vi "App - temperature sweep P1.vi"() -> ()   [LabVIEW 2014]
uses:
  C:/Users/riggslab/Desktop/Paula/maglab ultrasound -- arkady_by20151113_modified/state.ctl
  C:/Users/riggslab/Desktop/Paula/maglab ultrasound -- arkady_by20151113_modified/Sample_Temperature_Source_Control.ctl
  save log.ctl
  RUS/Controls/Sweep settings.ctl
  RUS/Controls/Lock-in DAQ settings.ctl
  File/Controls/Save data settings.ctl
  File/Controls/File formats.ctl
  C:/Users/riggslab/Desktop/Paula/maglab ultrasound -- arkady_by20151113_modified/ITC Panel.ctl
  gas flow controller control.ctl
  gas flow control - progress.ctl
  alarm clock control.ctl
  temperature indicator.ctl
  adaptive sweep UI controls.ctl
  next chunk -- algorithm.ctl
  time in gamma mode control.ctl
  Set Temperature PID - Control.ctl
  Scott -- strain -- strain sweep control.ctl
  FSU/ScottRiggs/Piezo2/voltage-wave-generator-parameters.ctl
  pair.ctl
  ctl -- name dispatcher -- action.ctl
  p9action control.ctl
  countdown control.ctl
  gas flow controller action.ctl
  C:/Users/riggslab/Desktop/Paula/maglab ultrasound -- arkady_by20151113_modified/itc 503 box - control.ctl
  Instruments/Neocera/Neocera Set Point Aproach.ctl
  file -- 9w path.vi
  Q - not nan -- real.vi
  Q - not nan and gtr than zero.vi
  switch - C.vi
  aggregator - ii - real.vi
  linear interpolation.vi
  <vilib>/Utility/libraryn.llb/Check if File or Folder Exists.vi
  file -- scan filename logic -- V1.vi
  <vilib>/Utility/file.llb/Write To Spreadsheet File.vi
  <vilib>/Utility/file.llb/Write To Spreadsheet File (string).vi
  <vilib>/regexp/Match Regular Expression.xnode
  Scott -- strain -- sweep parameter action.ctl
panel:
  in  "sweep folder path":path=path "D:/Technique/RUS/URuSi/DU45-325/2_cooling"
  in  "Tab: everything":T1(tab)=enum."temperature" caption="Tab Control"
  in  "Tab: RUS controls":T2(tab)
  in  "RUS settings":enum32{"main", "save and staff"}(tab)
  in  "adaptive sweep settings":T3={"time gap (min) "=0.0, "Bypass error dialog"=TRUE, "range factor"=1.35, "min gamma(kHz)"=0.005, "max step(Hz)"=1500.0, "min step(Hz)"=0.001, "save freq units"=enum."kHz", "Zero signal?"=FALSE, "time in Gamma --OK"=TRUE, "scan mode"=enum."peak position is known", "power control mode "=enum."none", "time-in-gamma mode"=enum."same for all"}
  in  "Lock-in DAQ settings":T6={"Lockin mode"=enum."NI-DAQ", "DAQmx Device"="Dev2", "SR Lockin"="GPIB0::10::INSTR", "Clock Multiplier"=64, "Low-pass filter"=enum."No filtering", "Ranges and couplings "=[{"Range"=2.5, "Coupling"=10106}], "Samples per read"=20, "Record IF"=FALSE, "Auto-phase"=FALSE} {"Ranges and couplings"."Coupling" items=["default"=-1, "RSE"=10083, "NRSE"=10078, "Differential"=10106, "Pseudodifferential"=12529]}
  in  "Fast sweep settings":T7={"Update rate (Hz)"=200.0, "Start F, Hz"=100000.0, "Stop F"=3500000.0, "Number of points"=7290, "Amplitude"=0.7, "Init&amplitude"=TRUE, "IF"=1000.0, "Time constant"=0.001} {"IF" format="%#_6p"; "Amplitude" min=0.0 max=2.5; "Number of points" format="%.0p"; "Stop F" format="%#_6p"; "Start F, Hz" format="%#_6p"; "Update rate (Hz)" format="%0.2f"}
  in  "Save data settings":T8={"Save data"=TRUE, "Data Root Path"=path "D:/Technique/RUS/URuSi/DU45-325/2_cooling", "File Prefix"="298.56700K_100_3500_0.70000V_0.00000T_Jul13-2015__11-06-01_", "File Format"=enum."BINARY", "Save column names"=FALSE, "File Comments"="\r\nColumns:Frequency\\tX\\tY\r\n    ITC Temp= 299.200000\r\n    LTC Temp= 0.000000\r\n          ITC_set=295.00000\r\n", "User/Prj"="<User Name/Project Description>"}
  out "sweep time  (min)":dbl=3.3333333333333335
  out "sweep time (sec)":i32=200
  out "kHz/second":dbl=17.0
  in  "RUS loop":bool=TRUE
  in  "RUS zeroed":bool
  in  "read AH every # sec":dbl=1.7
  in  "plot":T10(ring)=enum."Capac vs Temp"
  out "temperature":dbl=198.969
  out "time(min)":dbl
  out "Capacitance":dbl=0.600435
  out "Loss":dbl=0.00206
  in  "save every # (min)":dbl=7.12
  in  "history length (min)":dbl=60.0
  in  "Sweep folder path":path=path "C:/data/RUS/Experiment/ProbeTest/cantilever/Hg1201-2-2/sweep1"
  in  "VISA - AH2500":refnum<visa-resource-name>="GPIB0::28::INSTR"
  in  "take cantilever reading":bool=TRUE
  out "Plot: capacitance":cluster{dbl[], dbl[]}[](graph)
  in  "plot lever  ?":bool
  in  "Strain Inner Tabs":enum32{"Other", "Main"}(tab)=enum."Main"
  in  "time gap (min)":dbl
  in  "strain sweep control":T11={"just in case"=TRUE, "Piezo Amplifier settings"={"Gain "=69.44, "offset (V)"=-50.0}, "voltage-parameters-IN"={"phase "=0.7853981633974483, "amplitude (V)"=2.8801843317972353, "offset (V)"=0.0, "time delay (sec)"=0.5, "period (sec)"=50.0, "shape"=enum."triangle"}, "Lockin Settings"=[{"Offset"=FALSE, "GPIB Address"=6}, {"Offset"=TRUE, "GPIB Address"=7}], "VISA address Agilent  IN"="GPIB0::22::INSTR", "number of iterations"=1.0, "Piezo sweep settings"={"max Piezo voltage (V) "=150.0, "min Piezo voltage (V)"=-50.0, "delay (sec)"=0.5, "period (sec)"=50.0, "shape"=enum."triangle"}}
  in  "Strain loop":bool
  in  "show plot pallets":bool
  in  "Tab: ITC controls":enum32{"display", "gas ", "progress"}(tab)
  in  "set  T target":T13(ring)=enum."set T -> ITC (oxford)"
  in  "Set Temperature PID":T14={"mode "=enum."bezier", "set temperature?"=FALSE, "Time(min)"=646.03001, "Temperature(K)"=251.5695804259867, "OK?"=TRUE, "interval(sec)"=3.1}
  in  "ITC panel":T15={"Locked"=TRUE, "Unlocked"=FALSE, "Remote"=FALSE, "Local"=TRUE, "in sweep"=FALSE, "start/stop sweep"=FALSE, "Sweep indicator"="NOT in sweep", "heater MANUAL"=TRUE, "heater AUTO"=FALSE, "ITC state"="X0A1C2S01H1L0\r", "gas MANUAL"=TRUE, "gas AUTO"=FALSE, "heater"=5.999, "gas flow %"=20.587} {"gas flow %" format="%.3g"; "heater" format="%.3g"}
  in  "itc box: set temperature to: value":dbl=295.0
  in  "set temperature to":bool
  in  "disable interaction with itc":T16(ring)
  in  "plot?":bool=TRUE
  in  "set heater to":bool
  in  "itc box: set heater to: value":dbl=7.0
  in  "gas flow controller":T17={"DOWN step (%)"=0.5, "below"=FALSE, "above"=FALSE, "check (min)"=3.0, "upper"=12.0, "lower"=5.0, "in range"=TRUE, "ramp step (%)"=0.1, "DOWN time (min)"=20.0, "UP time (min)"=20.0, "UP step (%)"=0.5, "set gas"=FALSE, "to"=20.0, "ramp UP"=FALSE, "ramp DOWN"=FALSE, "idle"=TRUE, "Control Gas"=TRUE, "state"=enum."normal", "ramp Up progress"={"(total # of ramp steps)"=5, "ramp time step (sec)"=240, "steps so far"=0, "state"=enum."normal"}, "ramp Down progress"={"(total # of ramp steps)"=5, "ramp time step (sec)"=240, "steps so far"=0, "state"=enum."normal"}, "last (min)"=1.4983333333333335, "heater"=5.9990000000000085, "gas, %"=20.587} {"last (min)" format="%3.3f"}
  out "ramp Down progress":T18={"(total # of ramp steps)"=5, "ramp time step (sec)"=240, "steps so far"=0, "state"=enum."normal"}
  out "ramp Up progress":T18={"(total # of ramp steps)"=5, "ramp time step (sec)"=240, "steps so far"=0, "state"=enum."normal"}
  in  "Tab: plots":enum32{"Plot:  gas/heater", "Plot: temperayre"}(tab)=enum."Plot: temperayre"
  out "Plot: heater/gas":cluster{dbl[], dbl[]}[](graph)
  out "Plot: temperature":cluster{dbl[], dbl[]}[](graph)
  in  "Tab: controls":enum32{"indicators", "counter", "boxes"}(tab)
  in  "temperature indicator panel":T19={"LTC T"=298.568, "ITC T"=296.823, "ITC Set T"=296.82, "LTC T slope, K/min"=-0.0031198686372143165, "heater i-average, V"=5.999000000000011, "heater slope, V/min"=1.6517122458476368e-14, "LTC T i-average, K"=298.56648412698405, "ITC T i-average, K"=-2.7308309131347598e-14, "gas"=0.0} {"ITC Set T" format="%.3g"; "ITC T" format="%.3g"; "LTC T" format="%.3g"; "gas" format="%.3g"; "ITC T i-average, K" format="%#.5f"; "LTC T i-average, K" format="%#.5f"; "heater i-average, V" format="%.3g"; "heater slope, V/min" format="%#.5f"; "LTC T slope, K/min" format="%#.5f"}
  in  "Tab : everything to zero":enum32{"Page 1", "Page 2"}(tab)
  in  "alarm":T20={"counter (min)"=0.0, "alarm"=FALSE, "start"=FALSE, "set (min)"=1600.0, "stop"=FALSE} {"set (min)" format="%_4f"; "counter (min)" format="%_4f"}
  in  "Tab : Overheat":enum32{"Page 1"}(tab)
  in  "Over heat Temperature":dbl=315.0
  in  "Overheat protection":bool
  in  "Overheat !!":bool
  in  "temperature boxes":T21={"LTC21 Address"="GPIB0::15::INSTR", "ITC503 Address"="GPIB0::1::1::INSTR", "ITC temperature"=296.823, "ITC set temperature"=296.82, "LTC temperature"=298.568, "heater"=5.999, "gas flow"=20.587, "P"=6.5, "D"=0.0, "I"=0.9, "ITC state"="", "nonzero temperature"=298.568, "Magn Field (T)"=0.0, "LakeShore340"="GPIB0::11::INSTR", "LS340 Adress"=11, "Sample Temperature Source"=enum."read T <- LakeShore 340", "Neocera sensor"=1}
  in  "PID timer":dbl(slide)=86.6820000000298 min=-85661543.0 max=2135380277.0 step=0.010000000000000002 scale=0.0..100.0 scale format="%#3_3f"
  out "PID OK":bool=TRUE
  out "PID":dbl[](array[numeric])=[9.448275387987417, 0.584305003790149, 0.1]
  out "PID temperature":dbl=296.823
  out "Uploading ...":bool
  in  "Tab : Upload Sweep table":enum32{"Page 1"}(tab)
  out "Sweep Rates , min/K":dbl[](array[numeric])=[12.0, -0.0, 0.0, 0.0, 0.0, 0.0, 0.0, 0.0, 0.0, 0.0, 0.0, 0.0, 0.0, 0.0, 0.0, 0.0]
  out "current set temperature":dbl=50.0
  in  "set temperature":dbl=295.0
  in  "new sweep table":dbl[][](array[numeric])=[[200.0, 1000.0, 0.0], [100.0, 500.0, 0.0], [0.0, 0.0, 0.0], [0.0, 0.0, 0.0], [0.0, 0.0, 0.0], [0.0, 0.0, 0.0], [0.0, 0.0, 0.0], [0.0, 0.0, 0.0], [0.0, 0.0, 0.0], [0.0, 0.0, 0.0], [0.0, 0.0, 0.0], [0.0, 0.0, 0.0], [0.0, 0.0, 0.0], [0.0, 0.0, 0.0], [0.0, 0.0, 0.0], [70.0, 0.0, 0.0]]
  in  "Read Sweep Table in the box":bool
  out "Sweep Table":dbl[][](array[numeric])=[[70.0, 240.0, 1000.0], [0.0, 0.0, 0.0], [0.0, 0.0, 0.0], [0.0, 0.0, 0.0], [0.0, 0.0, 0.0], [0.0, 0.0, 0.0], [0.0, 0.0, 0.0], [0.0, 0.0, 0.0], [0.0, 0.0, 0.0], [0.0, 0.0, 0.0], [0.0, 0.0, 0.0], [0.0, 0.0, 0.0], [0.0, 0.0, 0.0], [0.0, 0.0, 0.0], [0.0, 0.0, 0.0], [70.0, 0.0, 0.0]]
  in  "upload new sweep table":bool
  out "index":dbl[][](array[numeric])=[[0.0, 1200.0, 0.0], [1.0, 1200.0, 0.0], [2.0, 500.0, 0.0], [3.0, 1399.0, 0.0], [4.0, 10.0, 1399.0], [5.0, 10.0, 1399.0], [6.0, 0.0, 0.0], [7.0, 0.0, 0.0], [8.0, 0.0, 0.0], [9.0, 0.0, 0.0], [10.0, 0.0, 0.0], [11.0, 0.0, 0.0], [12.0, 0.0, 0.0], [13.0, 0.0, 0.0], [14.0, 0.0, 0.0], [15.0, 0.0, 0.0]]
  out "date string Array":string[](array[string])=["Fri, Mar 07, 2014   :   11:06 AM", "Fri, Mar 07, 2014   :   3:06 PM"]
  in  "Rates , min/K":dbl[](array[numeric])=[12.0, -0.0, 0.0, 0.0, 0.0, 0.0, 0.0, 0.0, 0.0, 0.0, 0.0, 0.0, 0.0, 0.0, 0.0, 0.0]
  in  "use":bool
  out "writing log to":string="E:\\data\\Ultrasound\\Experiment\\ProbeTest\\Birdcage\\saphire-test\\1_test\\itc_log\\Stability_101113.dat"
  out "log line":string="time=Oct11,2013__13:45:08\tLTC=0.00000\tITC=0.00000\t ITC_set=0.00000\t\t filename=300.00000K_200_1000_2.10000V_0.00000T_Oct11-2013__13-45-08_101113.dat\t"
  out "saving log to":string
  out "saving sweep table to":string
  in  "save log":T23={"file path"=path "E:/data/Ultrasound/Experiment/ProbeTest/Birdcage/saphire-test/1_test", "Save log?"=TRUE, "every # of sec"=64}
  in  "set gas % to":dbl=10.0
  out "9ctl OK":bool
  out "minutes":dbl=1.4983333333333335
  out "milliseconds per cycle":u32=3100
  out "seconds per cycle":dbl=3.1
  out "file name prefix":string="298.56700K_100_3500_0.70000V_0.00000T_Jul13-2015__11-06-01_"
  out "x-y":dbl=37.2
  out "seconds":dbl=89.9
  in  "error in":errorcluster
  # "1. Make sure the correct experiment is hard-wired in the block diagram.\n2. Folder with 9w sub-folder. \n3. Reset ctl_set_temperature_TIMER file to 0.\n4. Set-up the ctl_set_temperature file."
  # "69.44"
  # "the paths are copied from \"data root path\" in the first page"
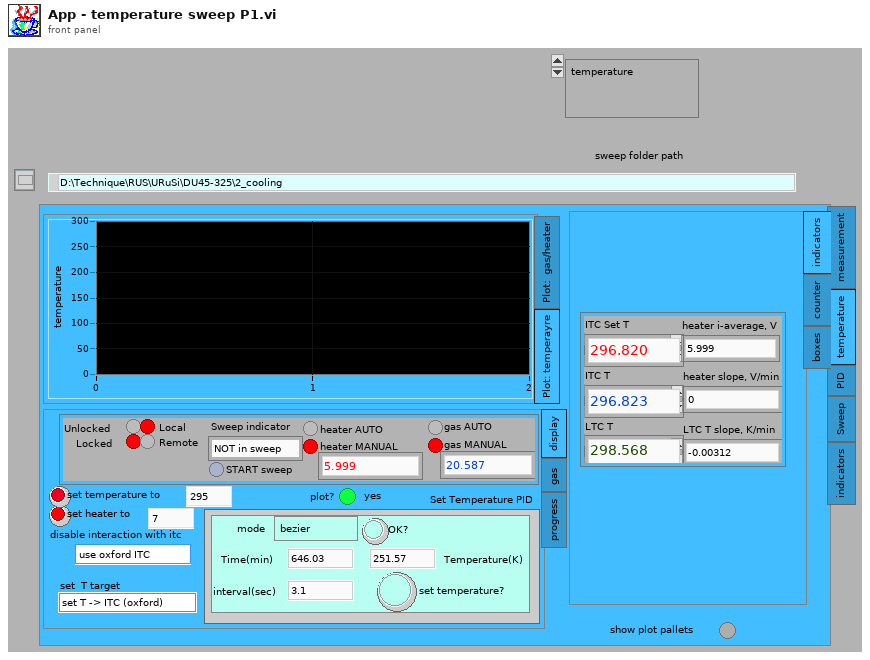
[diagram p1: front panel]
types:
  T1 = enum32{"measurement", "temperature", "PID", "Sweep", "indicators"}
  T2 = enum32{"Resonant Ultrasound", "Cantilever", "Strain"}
  T3 = typedef "adaptive sweep UI controls.ctl" = cluster{"time gap (min) ":dbl, "Bypass error dialog":bool, "range factor":dbl, "min gamma(kHz)":dbl, "max step(Hz)":dbl, "min step(Hz)":dbl, "save freq units":enum16{"kHz", "Hz"}, "Zero signal?":bool, "time in Gamma --OK":bool, "scan mode":T4, "power control mode ":enum16{"power vs Temp", "power vs Time", "none"}, "time-in-gamma mode":T5}
  T4 = typedef "next chunk -- algorithm.ctl" = enum16{"peak position is known", "uniform", "predictive"}
  T5 = typedef "time in gamma mode control.ctl" = enum16{"same for all", "each one different", "uniform scan"}
  T6 = typedef "Lock-in DAQ settings.ctl" = cluster{"Lockin mode":enum16{"SRS", "NI-DAQ"}, "DAQmx Device":tag, "SR Lockin":refnum<visa-resource-name>, "Clock Multiplier":i32, "Low-pass filter":enum16{"No filtering", "Butterworth", "Bessel"}, "Ranges and couplings ":cluster{"Range":dbl, "Coupling":i32}[], "Samples per read":i32, "Record IF":bool, "Auto-phase":bool}
  T7 = typedef "Sweep settings.ctl" = cluster{"Update rate (Hz)":dbl, "Start F, Hz":dbl, "Stop F":dbl, "Number of points":i32, "Amplitude":dbl, "Init&amplitude":bool, "IF":dbl, "Time constant":dbl}
  T8 = typedef "Save data settings.ctl" = cluster{"Save data":bool, "Data Root Path":path, "File Prefix":string, "File Format":T9, "Save column names":bool, "File Comments":string, "User/Prj":string}
  T9 = typedef "File formats.ctl" = enum16{"TDMS", "ASCII", "BINARY"}
  T10 = enum16{"Capac vs Time", "Capac vs Temp", "Loss  vs Time", "Loss vs Temp", "Delta Cap vs Temp"}
  T11 = typedef "Scott -- strain -- strain sweep control.ctl" = cluster{"just in case":bool, "Piezo Amplifier settings":cluster{"Gain ":dbl, "offset (V)":dbl}, "voltage-parameters-IN":T12, "Lockin Settings":cluster{"Offset":bool, "GPIB Address":i16}[], "VISA address Agilent  IN":refnum<visa-resource-name>, "number of iterations":dbl, "Piezo sweep settings":cluster{"max Piezo voltage (V) ":dbl, "min Piezo voltage (V)":dbl, "delay (sec)":dbl, "period (sec)":dbl, "shape":enum16{"triangle", "sine", "none"}}}
  T12 = typedef "voltage-wave-generator-parameters.ctl" = cluster{"phase ":dbl, "amplitude (V)":dbl, "offset (V)":dbl, "time delay (sec)":dbl, "period (sec)":dbl, "shape":enum16{"triangle", "sine", "none"}}
  T13 = enum16{"set T -> LTC (neocera)", "set T -> ITC (oxford)"}
  T14 = typedef "Set Temperature PID - Control.ctl" = cluster{"mode ":enum16{"bezier", "sine wave"}, "set temperature?":bool, "Time(min)":dbl, "Temperature(K)":dbl, "OK?":bool, "interval(sec)":dbl}
  T15 = typedef "ITC Panel.ctl" = cluster{"Locked":bool, "Unlocked":bool, "Remote":bool, "Local":bool, "in sweep":bool, "start/stop sweep":bool, "Sweep indicator":string, "heater MANUAL":bool, "heater AUTO":bool, "ITC state":string, "gas MANUAL":bool, "gas AUTO":bool, "heater":dbl, "gas flow %":dbl}
  T16 = enum16{"use oxford ITC", "do not use oxford ITC"}
  T17 = typedef "gas flow controller control.ctl" = cluster{"DOWN step (%)":dbl, "below":bool, "above":bool, "check (min)":dbl, "upper":dbl, "lower":dbl, "in range":bool, "ramp step (%)":dbl, "DOWN time (min)":dbl, "UP time (min)":dbl, "UP step (%)":dbl, "set gas":bool, "to":dbl, "ramp UP":bool, "ramp DOWN":bool, "idle":bool, "Control Gas":bool, "state":enum16{"normal", "ramp up", "ramp down"}, "ramp Up progress":T18, "ramp Down progress":T18, "last (min)":dbl, "heater":dbl, "gas, %":dbl}
  T18 = typedef "gas flow control - progress.ctl" = cluster{"(total # of ramp steps)":i32, "ramp time step (sec)":i32, "steps so far":i32, "state":enum16{"normal", "ramp up", "ramp down"}}
  T19 = typedef "temperature indicator.ctl" = cluster{"LTC T":dbl, "ITC T":dbl, "ITC Set T":dbl, "LTC T slope, K/min":dbl, "heater i-average, V":dbl, "heater slope, V/min":dbl, "LTC T i-average, K":dbl, "ITC T i-average, K":dbl, "gas":dbl}
  T20 = typedef "alarm clock control.ctl" = cluster{"counter (min)":dbl, "alarm":bool, "start":bool, "set (min)":dbl, "stop":bool}
  T21 = typedef "state.ctl" = cluster{"LTC21 Address":refnum<visa-resource-name>, "ITC503 Address":refnum<visa-resource-name>, "ITC temperature":dbl, "ITC set temperature":dbl, "LTC temperature":dbl, "heater":dbl, "gas flow":dbl, "P":dbl, "D":dbl, "I":dbl, "ITC state":string, "nonzero temperature":dbl, "Magn Field (T)":dbl, "LakeShore340":refnum<visa-resource-name>, "LS340 Adress":i16, "Sample Temperature Source":T22, "Neocera sensor":i32}
  T22 = typedef "Sample_Temperature_Source_Control.ctl" = enum16{"read T <- LakeShore 340", "read T <- Neocera"}
  T23 = typedef "save log.ctl" = cluster{"file path":path, "Save log?":bool, "every # of sec":i32}
  T24 = typedef "pair.ctl" = cluster{"num":i32, "bool":bool, "string":string}
  T25 = typedef "ctl -- name dispatcher -- action.ctl" = enum16{"peak frequency", "peak frequency DUMP", "peak gamma DUMP", "peak gamma", "peak frequency TEST", "peak gamma TEST", "ultrasonic power", "time in gamma", "set temperature ", "set temperature timer", "peak default gamma", "last scan file", "peak freq gamma TEST", "peak NAMES", "errors", "P_I_D", "P", "I", "D", "power vs time", "power vs time TIMER", "void", "power log", "set temperature - SINE", "itc ltc log", "peak - time in gamma"}
  T26 = typedef "Scott -- strain -- sweep parameter action.ctl" = enum16{"calculate gain and stuff", "none"}
  T27 = typedef "file -- scan filename.ctl" = cluster{"mmddyy (str)":string, "counter (str)":string, "to F (kHz)":dbl, "from F (kHz)":dbl, "temperature (K)":dbl, "date/time string":string, "time stamp":timestamp, "base name":string, "temperature (str)":string, "from F (str)":string, "to F (str)":string, "format":enum16{"no date string", "with date string"}, "power (V)":dbl, "power (str) ":string, "Magn Field (T)":dbl, "Magn Field (str)":string}
  T28 = cluster{"temperature array":dbl[], "delta capacitance array":dbl[]}
  T29 = cluster{"temperature array":dbl[], "delta capacitance array":dbl[]}[]
  T30 = typedef "p9action control.ctl" = enum16{"init", "check", "reset", "log", "message", "change path"}
  T31 = typedef "countdown control.ctl" = enum16{"check", "start", "reset cont", "stop", "reset once"}
  T32 = typedef "gas flow controller action.ctl" = enum16{"check", "force UP", "stop UP/DOWN", "force DOWN", "init", "set gas to", "turn off", "turn on", "idle", "update parameters", "parse", "set gas"}
  T33 = typedef "itc 503 box - control.ctl" = enum16{"heater manual and zero", "heater auto", "upload D", "upload I", "upload P", "shut off", "init", "read sweep table", "disable", "enable", "read state", "set gas to", "stop sweep", "start sweep", "test", "set temperature to", "write sweep table", "-void", "set heater to"}
  T34 = enum16{"table to rates", "rates to table", "other"}
  T35 = enum16{"parse", "start sweep", "stop sweep", "heater auto", "heater manual", "set heater"}
  T36 = enum8{"Enabled", "Disabled", "Disabled and Grayed Out"}
  T37 = typedef "Neocera Set Point Aproach.ctl" = enum16{"Instant", "Ramp"}
  T38 = typedef "itc 503 box state.ctl" = cluster{"ITC503 Address":refnum<visa-resource-name>, "ITC temperature":dbl, "ITC set temperature":dbl, "heater":dbl, "gas flow":dbl, "P":dbl, "D":dbl, "I":dbl, "ITC state":string, "nonzero temperature":dbl, "Magn Field (T)":dbl}
  T39 = enum16{"check", "force UP", "stop UP/DOWN", "force DOWN", "init", "set gas to", "turn off", "turn on", "update parameters"}
  T40 = enum32{"Page Enabled", "Page Disabled", "Page Disabled & Grayed"}
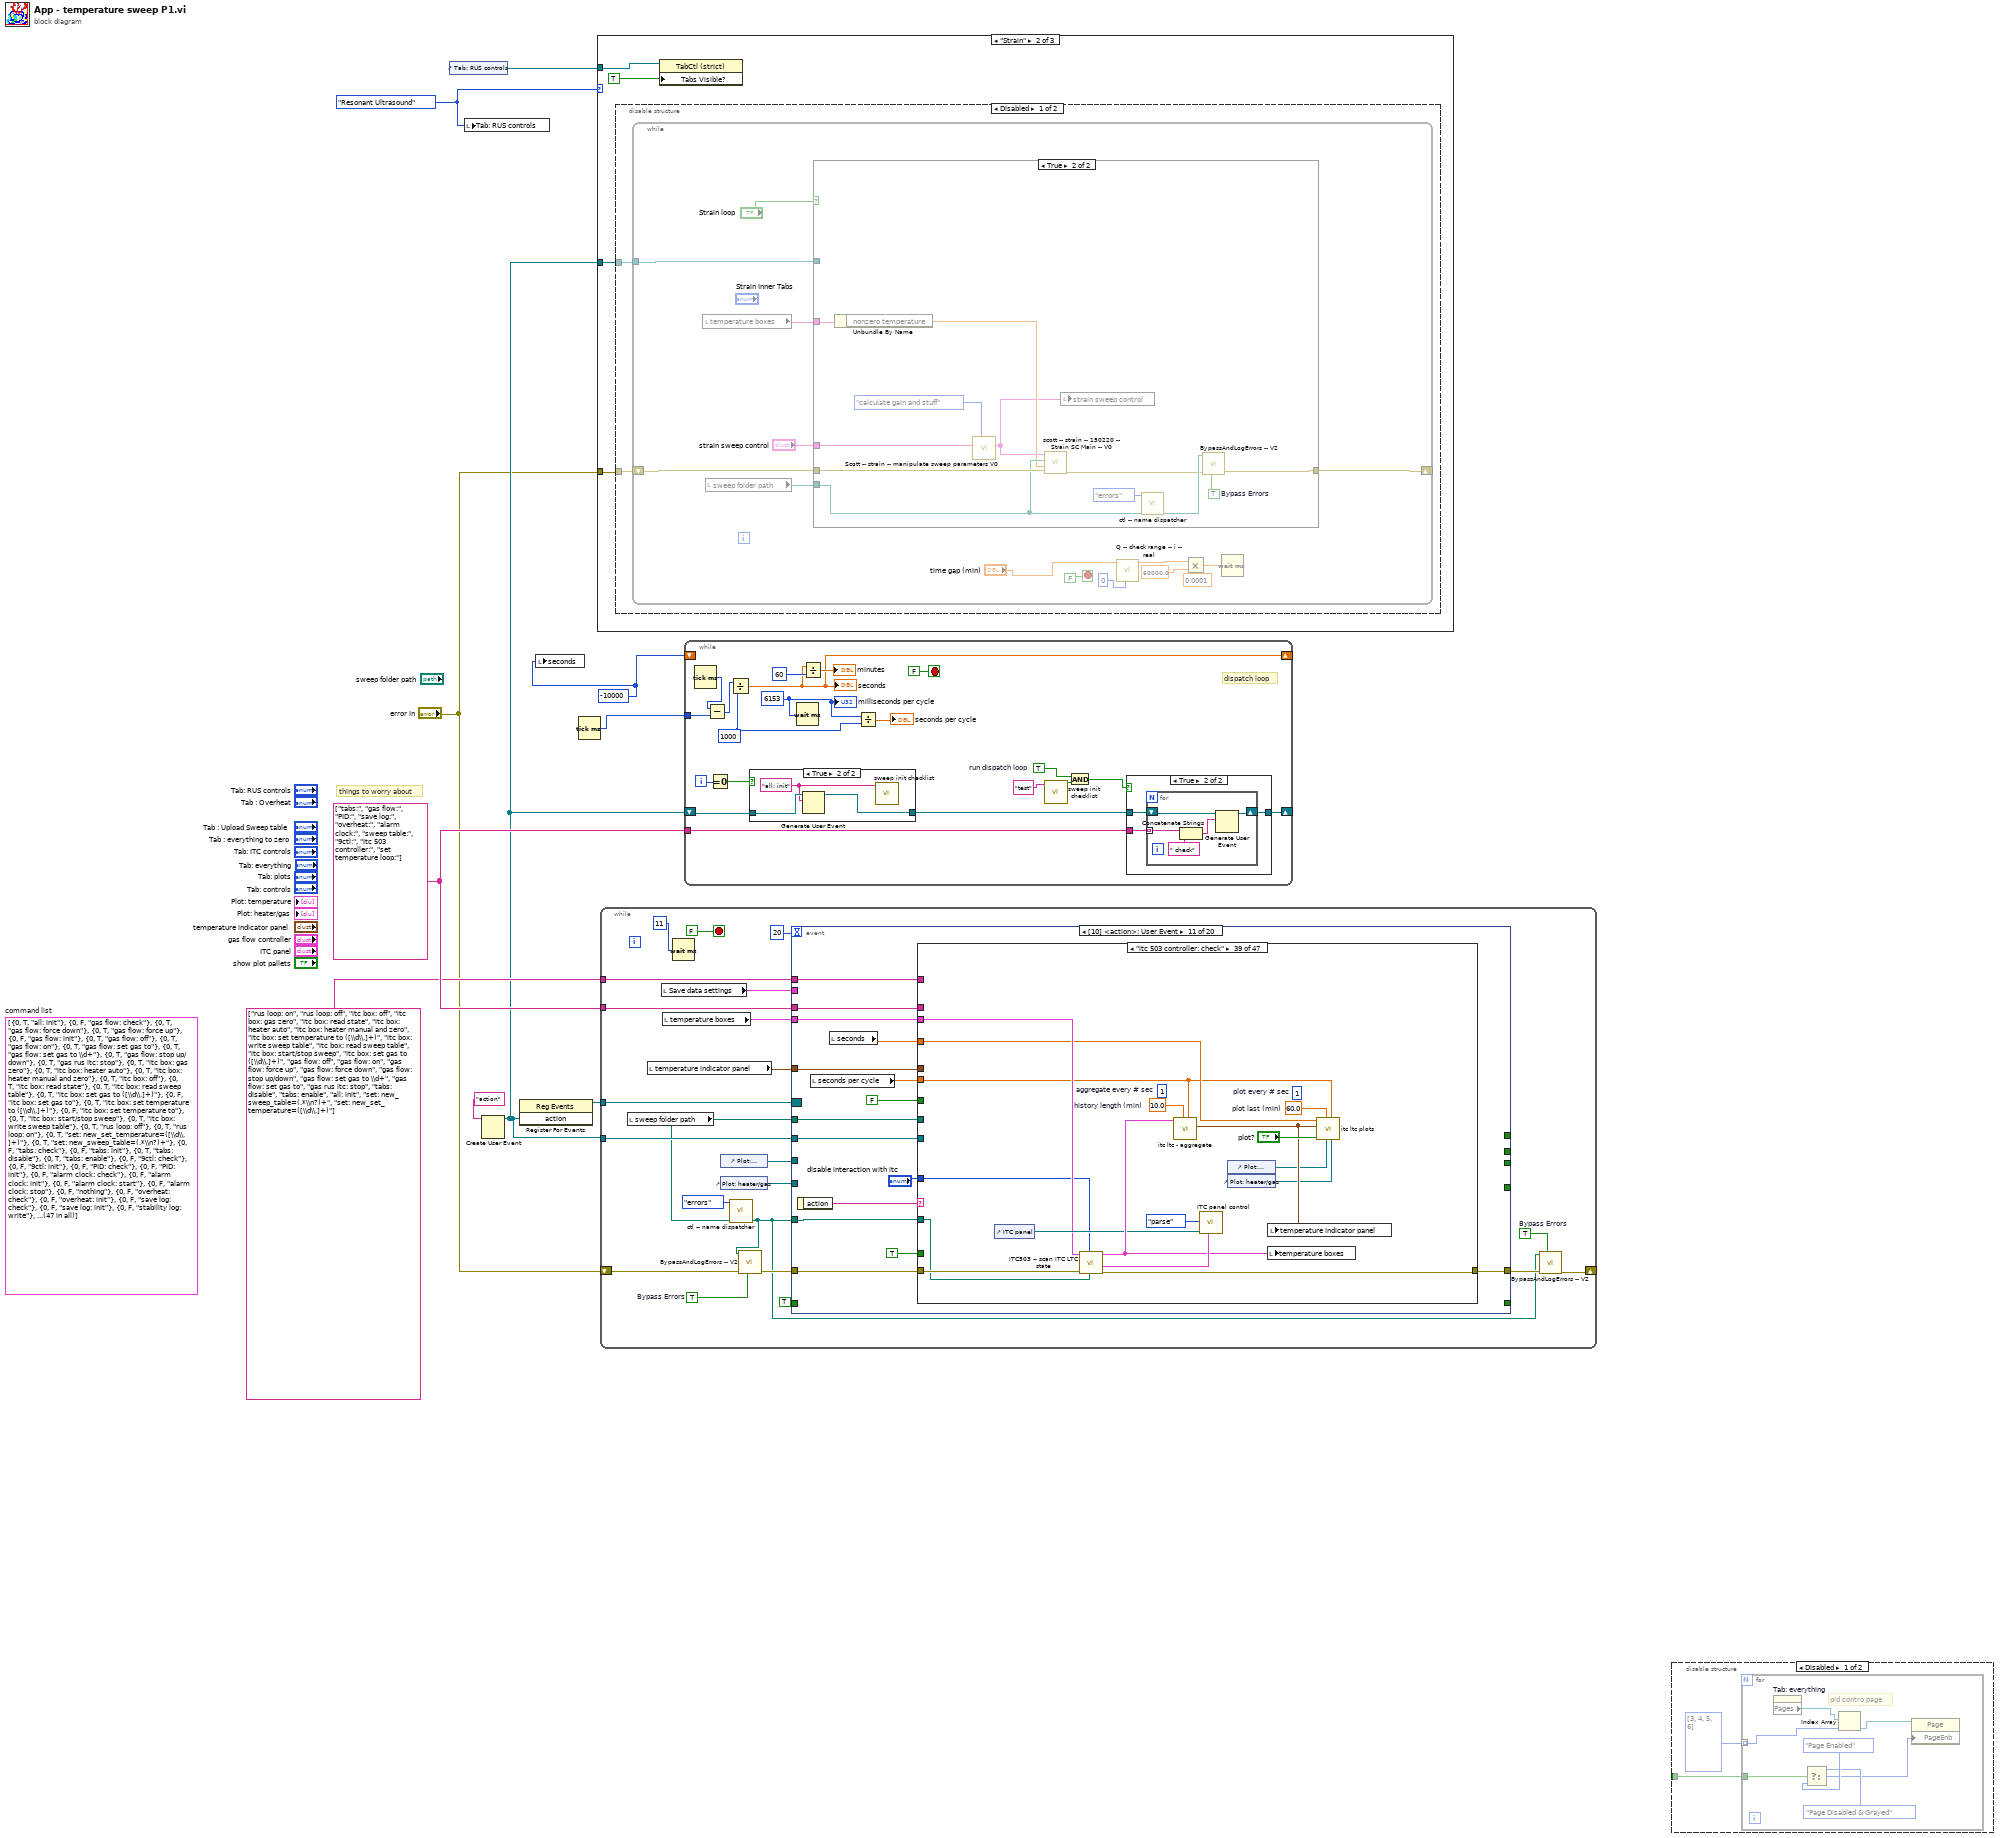
[diagram p0: block diagram]
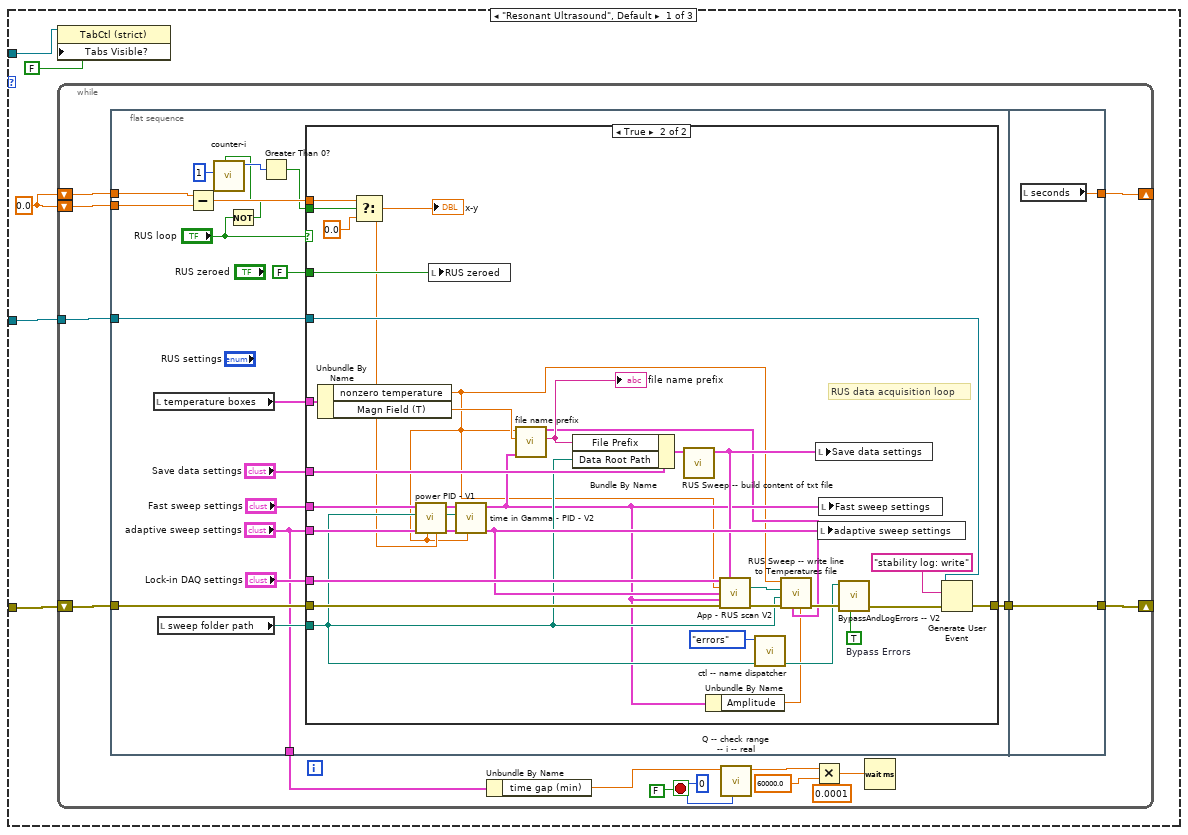
[diagram p2: hidden frame]
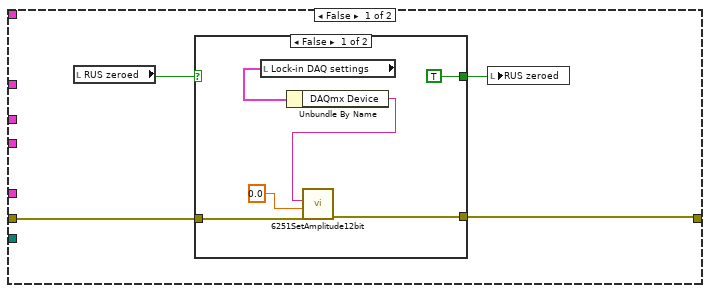
[diagram p3: hidden frame]
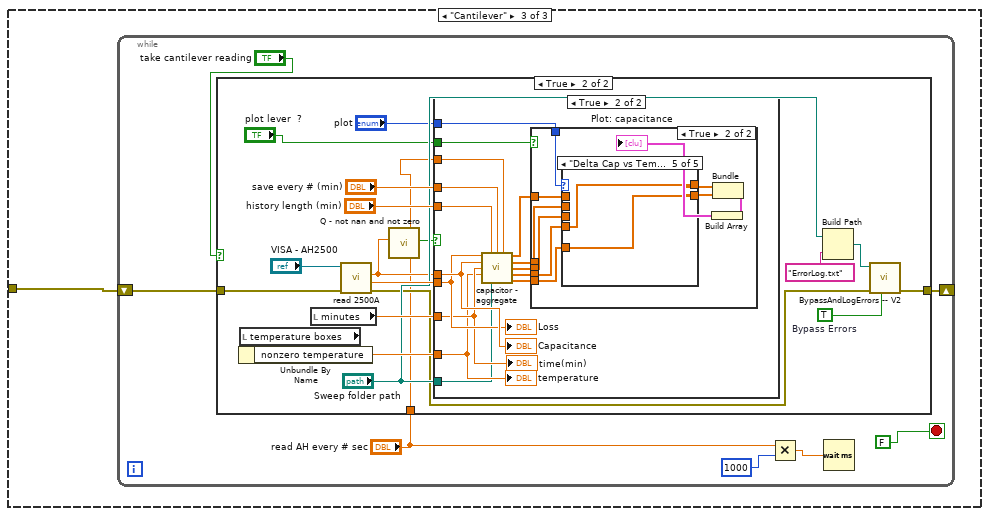
[diagram p7: hidden frame]
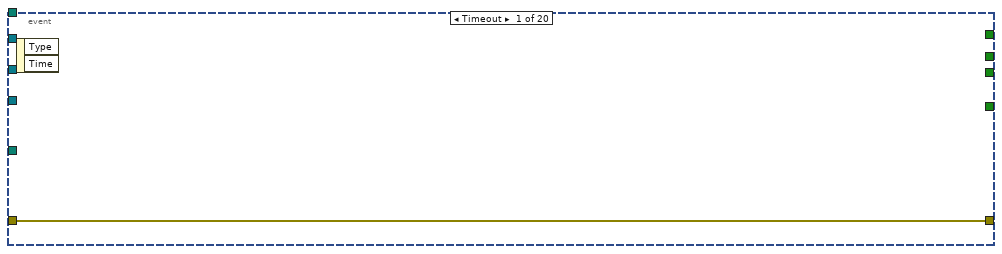
[diagram p16: hidden frame]
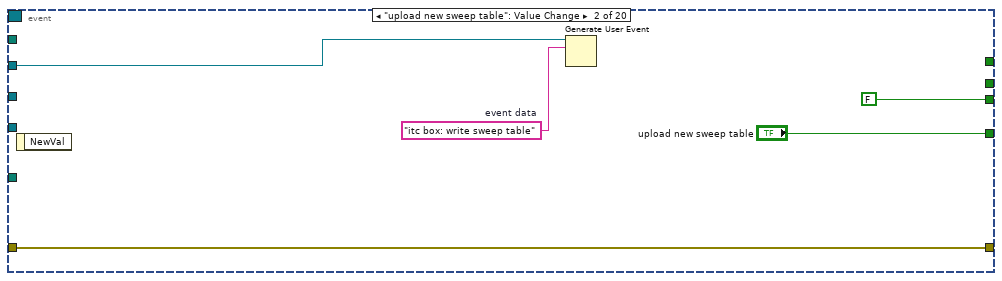
[diagram p17: hidden frame]
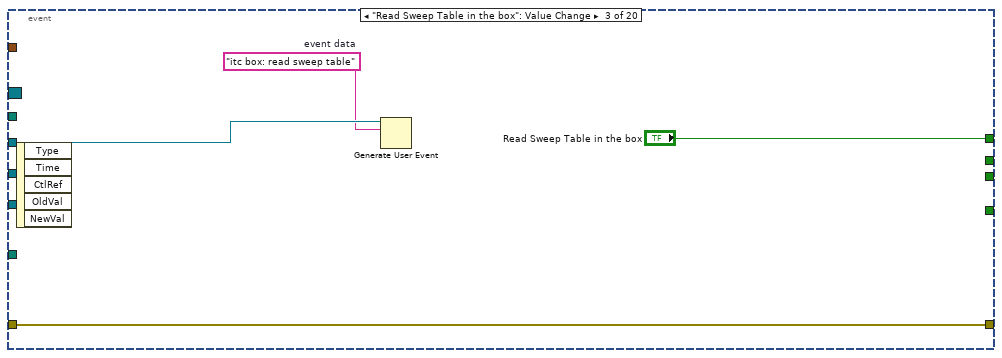
[diagram p18: hidden frame]
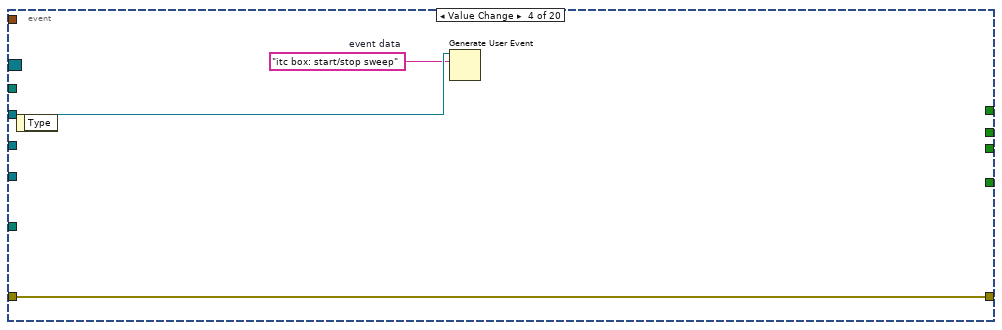
[diagram p19: hidden frame]
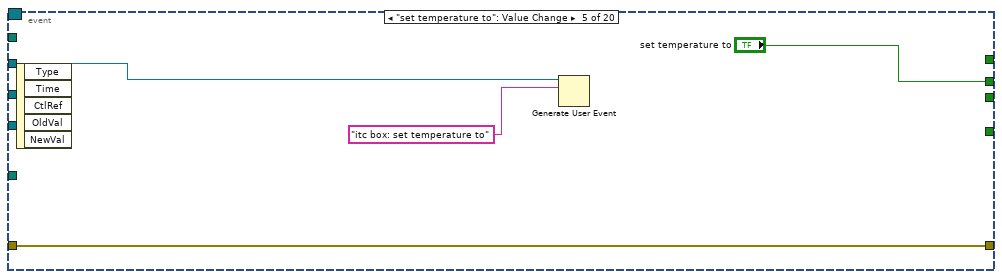
[diagram p20: hidden frame]
diagram:
  w2 = -10000 ("y")
  w1 = T2."Resonant Ultrasound" ("Tab: RUS controls")
  (unwired) T24[] [{"num"=0, "bool"=TRUE, "string"="all: init"}, {"num"=0, "bool"=FALSE, "string"="gas flow: check"}, {"num"=0, "bool"=TRUE, "string"="gas flow: force down"}, {"num"=0, "bool"=TRUE, "string"="gas flow: force up"}, {"num"=0, "bool"=FALSE, "string"="gas flow: init"}, {"num"=0, "bool"=TRUE, "string"="gas flow: off"}, {"num"=0, "bool"=TRUE, "string"="gas flow: on"}, {"num"=0, "bool"=TRUE, "string"="gas flow: set gas to"}, {"num"=0, "bool"=TRUE, "string"="gas flow: set gas to \\d+"}, {"num"=0, "bool"=TRUE, "string"="gas flow: stop up/down"}, {"num"=0, "bool"=TRUE, "string"="gas rus itc: stop"}, {"num"=0, "bool"=TRUE, "string"="itc box: gas zero"}, {"num"=0, "bool"=TRUE, "string"="itc box: heater auto"}, {"num"=0, "bool"=TRUE, "string"="itc box: heater manual and zero"}, {"num"=0, "bool"=TRUE, "string"="itc box: off"}, {"num"=0, "bool"=TRUE, "string"="itc box: read state"}, {"num"=0, "bool"=TRUE, "string"="itc box: read sweep table"}, {"num"=0, "bool"=TRUE, "string"="itc box: set gas to ([\\d\\.]+)"}, {"num"=0, "bool"=FALSE, "string"="itc box: set gas to"}, {"num"=0, "bool"=TRUE, "string"="itc box: set temperature to ([\\d\\.]+)"}, {"num"=0, "bool"=FALSE, "string"="itc box: set temperature to"}, {"num"=0, "bool"=TRUE, "string"="itc box: start/stop sweep"}, {"num"=0, "bool"=TRUE, "string"="itc box: write sweep table"}, {"num"=0, "bool"=TRUE, "string"="rus loop: off"}, {"num"=0, "bool"=TRUE, "string"="rus loop: on"}, {"num"=0, "bool"=TRUE, "string"="set: new_set_temperature=([\\d\\.]+)"}, {"num"=0, "bool"=TRUE, "string"="set: new_sweep_table=(.*\\n?)+"}, {"num"=0, "bool"=FALSE, "string"="tabs: check"}, {"num"=0, "bool"=FALSE, "string"="tabs: init"}, {"num"=0, "bool"=TRUE, "string"="tabs: disable"}, {"num"=0, "bool"=TRUE, "string"="tabs: enable"}, {"num"=0, "bool"=FALSE, "string"="9ctl: check"}, {"num"=0, "bool"=FALSE, "string"="9ctl: init"}, {"num"=0, "bool"=FALSE, "string"="PID: check"}, {"num"=0, "bool"=FALSE, "string"="PID: init"}, {"num"=0, "bool"=FALSE, "string"="alarm clock: check"}, {"num"=0, "bool"=FALSE, "string"="alarm clock: init"}, {"num"=0, "bool"=FALSE, "string"="alarm clock: start"}, {"num"=0, "bool"=FALSE, "string"="alarm clock: stop"}, {"num"=0, "bool"=FALSE, "string"="nothing"}, {"num"=0, "bool"=FALSE, "string"="overheat: check"}, {"num"=0, "bool"=FALSE, "string"="overheat: init"}, {"num"=0, "bool"=FALSE, "string"="save log: check"}, {"num"=0, "bool"=FALSE, "string"="save log: init"}, {"num"=0, "bool"=FALSE, "string"="stability log: write"}, {"num"=0, "bool"=FALSE, "string"="sweep table: init"}, {"num"=0, "bool"=FALSE, "string"="sweep table: check"}]  # command list
  w8 = string[] ["tabs:", "gas flow:", "PID:", "save log:", "overheat:", "alarm clock:", "sweep table:", "9ctl:", "itc 503 controller:", "set temperature loop:"]
  # "things to worry about"
  n1 = control-ref of="Tab: RUS controls"() -> (w6:refnum<vi>)
  n2 = local write "Tab: RUS controls"(w1) -> ()
  n3 = Create User Event(user event datatype="action" ("action")) -> (user event=w5:refnum<user-event>)  [unwired: 1 in, 1 out]
  n4 = register-events(w5) -> (reference out=w10:refnum<event-registration>)  [unwired: 2 in, 1 out]
  n5 = local write "seconds"(w2) -> ()
  n6 = Tick Count (ms)() -> (millisecond timer value=w3:u32)
  n7 = case shown="\"Strain\"" w1 {
    tunnel: "error in" -> [w15 w98 w127]
    tunnel: w5 -> [w14 w97 _]
    tunnel: w6 -> [w12 w95 _]
    frame "Resonant Ultrasound", Default {
      w11 = 0.0
      n8 = property class="TabCtl (strict)"(reference=w12, "Tabs Visible?"=FALSE) -> ()  [unwired: 1 in, 2 out]
      n9 = while {
        shift-right: [w26] -> _
        shift-left: w15 -> [w29]
        tunnel: w14 -> [w24]
        shift-right: [w16] -> _
        shift-left: w11 -> [w19]
        shift-left: w11 -> [w18]
        stop <- FALSE stop-if-true
        (unwired) 0.0001
        n10 = flat-sequence {
          tunnel: w29 -> [w47]
          tunnel: w24 -> [w45]
          tunnel: ["adaptive sweep settings"] -> w21
          tunnel: w19 -> [w37]
          tunnel: w18 -> [w30]
          tunnel: [w46] -> w17
          tunnel: [w94] -> w26
          tunnel: w17 -> [w94]
          tunnel: [w93] -> w16
          frame #0 {
            n11 = local read "temperature boxes"() -> (w41:T21)
            n12 = local read "sweep folder path"() -> (w43:path)
            n13 = Subtract(x=w30, y=w37) -> (x-y=w36:dbl)
            n14 = Not(x="RUS loop") -> (.not. x?=w31:bool)
            n15 = call "counter-i.vi"("init ?"=w31, "cricket interval"=1) -> ("tic"=w34:i32)  [unwired: 8 in, 1 out]
            n16 = Greater Than 0?(x=w34) -> (x > 0?=w33:bool)
            n17 = case shown="True" "RUS loop" {
              tunnel: [w50 w83] -> w46
              tunnel: w47 -> [w51 w86]
              tunnel: w45 -> [_ w85]
              tunnel: FALSE ("frequency  format") -> [_ w81]
              tunnel: w43 -> [_ w69]
              tunnel: "Save data settings" -> [_ w77]
              tunnel: w41 -> [_ w76]
              tunnel: "Fast sweep settings" -> [_ w75]
              tunnel: "Lock-in DAQ settings" -> [_ w74]
              tunnel: "adaptive sweep settings" -> [_ w73]
              tunnel: w36 -> [_ w63]
              tunnel: w33 -> [_ w64]
              frame False {
                n18 = local read "RUS zeroed"() -> (w49:bool)
                n19 = case shown="False" w49 {
                  selector: w49 -> [_ w59]
                  tunnel: w51 -> [w56 w58]
                  tunnel: [w55 w58] -> w50
                  tunnel: [TRUE ("set amplitude to zero \nat end of every sweep") w59] -> w48
                  frame False {
                    n20 = local read "Lock-in DAQ settings"() -> (w54:T6)
                    n21 = Unbundle By Name(w54) -> ("DAQmx Device"=w53:tag)
                    n22 = call "6251SetAmplitude12bit.vi"("error in (no error)"=w56, "0 to 2.1 VRMS"=0.0, "DAQmx Device Name"=w53) -> ("error out"=w55:errorcluster)  [unwired: 8 out]
                  }
                  frame True {
                  }
                }
                n23 = local write "RUS zeroed"(w48) -> ()
              }
              frame True {
                w89 = TRUE  # Bypass Errors
                # "RUS data acquisition loop"
                n24 = Unbundle By Name(w76) -> ("nonzero temperature"=w60:dbl, "Magn Field (T)"=w61:dbl)
                n25 = Select(t=w63, s=w64, f=0.0) -> (s? t:f=w65:dbl)
                "x-y" <- w65
                n26 = call "power PID - V1.vi"("delta time(sec)"=w65, "nonzero temperature"=w60, "adaptive sweep settings"=w73, "sweep folder path"=w69, "Fast sweep settings"=w75) -> ("adaptive sweep settings OUT"=w72:T3, "Fast sweep settings out"=w80:T7)  [unwired: 3 in, 2 out]
                n27 = local write "RUS zeroed"(w81) -> ()
                n28 = call "time in Gamma - PID - V2.vi"("nonzero temperature"=w60, "adaptive sweep settings"=w72, "sweep folder path"=w69, "Fast sweep settings"=w80) -> ("adaptive sweep settings OUT"=w71:T3, "Fast sweep settings out"=w68:T7)  [unwired: 4 in, 2 out]
                n29 = call "file name prefix.vi"("Fast sweep settings"=w68, "Magn Field (T)"=w61, "temperature"=w60) -> ("file name prefix"=w90:string, "filename cluster OUT"=w67:T27)  [unwired: 5 in, 2 out]
                "file name prefix" <- w90
                n30 = Bundle By Name(cluster=w77, "File Prefix"=w90, "Data Root Path"=w69) -> (w91:T8)
                n31 = call "RUS Sweep -- build content of txt file.vi"("Save data settings"=w91) -> ("Save data settings out"=w70:T8)  [unwired: 9 in, 1 out]
                n32 = Unbundle By Name(w68) -> ("Amplitude"=w66:dbl)
                n33 = call "App - RUS scan V2.vi"("Lock-in DAQ settings"=w74, "Save data settings"=w70, "temperature"=w60, "sweep settings"=w71, "Fast swep settings"=w68, "error in (no error)"=w86) -> ("Actual file path"=w92:path, "error out"=w87:errorcluster)  [unwired: 8 in]
                n34 = call "ctl -- name dispatcher.vi"("sweep folder path"=w69, "ctl name dispatch"=ctl_--_name_dispatcher_--_action."errors" ("ctl kind")) -> ("file path"=w78:path)  [unwired: 7 in, 2 out]
                n35 = call "RUS Sweep -- write line to Temperatures file.vi"("voltage"=w66, "filename cluster OUT"=w67, "error in"=w87, "sweep folder path"=w69, "file path"=w92, "LTC Temperature"=w60) -> ("error out"=w88:errorcluster)  [unwired: 5 in]
                n36 = local write "Save data settings"(w70) -> ()
                n37 = local write "adaptive sweep settings"(w71) -> ()
                n38 = local write "Fast sweep settings"(w68) -> ()
                n39 = call "BypassAndLogErrors -- V2.vi"("Bypass Errors"=w89, "error in (no error)"=w88, "Log File Path"=w78) -> ("error out"=w82:errorcluster)  [unwired: 8 in]
                n40 = Generate User Event(user event=w85, event data cluster="stability log: write" ("name or relative path"), error in=w82) -> (error out=w83:errorcluster)  [unwired: 1 in, 1 out]
              }
            }
          }
          frame #1 {
            n41 = local read "seconds"() -> (w93:dbl)
          }
        }
        n42 = Unbundle By Name(w21) -> ("time gap (min)"=w20:dbl)
        n43 = call "Q -- check range -- i -- real.vi"("lower"=0, "number"=w20) -> ("number in range"=w22:dbl)  [unwired: 7 in, 2 out]
        n44 = Multiply(x=w22, y=60000.0) -> (x*y=w28:dbl)
        n45 = Wait (ms)(milliseconds to wait=w28) -> ()  [unwired: 1 out]
      }
    }
    frame "Strain" {
      n46 = disable-structure shown="Disabled" {
        disable-tunnel: w98 -> [w100 _]
        disable-tunnel: w97 -> [w99 _]
        frame Disabled {
          n47 = while {
            shift-right: [w110] -> _
            shift-left: w100 -> [w113]
            tunnel: w99 -> [w108]
            stop <- FALSE stop-if-true
            (unwired) 0.0001
            n48 = local read "temperature boxes"() -> (w103:T21)
            n49 = local read "sweep folder path"() -> (w104:path)
            n50 = case shown="True" "Strain loop" {
              tunnel: [w114 w122] -> w110
              tunnel: w113 -> [w114 w121]
              tunnel: w108 -> [_ _]
              tunnel: w104 -> [_ w119]
              tunnel: w103 -> [_ w123]
              tunnel: "strain sweep control" -> [_ w117]
              frame False {
              }
              frame True {
                w126 = TRUE  # Bypass Errors
                n51 = Unbundle By Name(w123) -> ("nonzero temperature"=w118:dbl)
                n52 = call "Scott -- strain -- manipulate sweep parameters V0.vi"("sweep parameters action"=Scott_--_strain_--_sweep_parameter_action."calculate gain and stuff", "strain sweep control"=w117) -> ("strain sweep control OUT"=w115:T11)  [unwired: 9 in]
                n53 = call "scott -- strain -- 150220 -- Strain SC Main -- V0.vi"("error in"=w121, "temperature"=w118, "sweep folder name"=w119, "strain sweep control"=w115) -> ("error out"=w120:errorcluster)  [unwired: 7 in]
                n54 = local write "strain sweep control"(w115) -> ()
                n55 = call "ctl -- name dispatcher.vi"("sweep folder path"=w119, "ctl name dispatch"=ctl_--_name_dispatcher_--_action."errors" ("ctl kind")) -> ("file path"=w124:path)  [unwired: 7 in, 2 out]
                n56 = call "BypassAndLogErrors -- V2.vi"("Bypass Errors"=w126, "error in (no error)"=w120, "Log File Path"=w124) -> ("error out"=w122:errorcluster)  [unwired: 8 in]
              }
            }
            n57 = call "Q -- check range -- i -- real.vi"("lower"=0, "number"="time gap (min)") -> ("number in range"=w106:dbl)  [unwired: 7 in, 2 out]
            n58 = Multiply(x=w106, y=60000.0) -> (x*y=w112:dbl)
            n59 = Wait (ms)(milliseconds to wait=w112) -> ()  [unwired: 1 out]
          }
        }
        frame Enabled {
        }
      }
      n60 = property class="TabCtl (strict)"(reference=w95, "Tabs Visible?"=TRUE) -> ()  [unwired: 1 in, 2 out]
    }
    frame "Cantilever" {
      n61 = while {
        shift-right: [w131] -> _
        shift-left: w127 -> [w132]
        stop <- FALSE ("Boolean") stop-if-true
        n62 = case shown="True" "take cantilever reading" {
          tunnel: w132 -> [w135 w143]
          tunnel: [w135 w141] -> w131
          tunnel: "read AH every # sec" -> [_ w136]
          frame False {
          }
          frame True {
            w147 = TRUE  # Bypass Errors
            n63 = local read "temperature boxes"() -> (w149:T21)
            n64 = Unbundle By Name(w149) -> ("nonzero temperature"=w148:dbl)
            n65 = local read "minutes"() -> (w150:dbl)
            n66 = call "read 2500A.vi"("error in (no error)"=w143, "VISA Resource Name"="VISA - AH2500") -> ("error out"=w142:errorcluster, "Loss"=w151:dbl, "Capacitance"=w140:dbl)  [unwired: 6 in, 1 out]
            n67 = call "Q - not nan and not zero.vi"("Numeric"=w140) -> ("Boolean"=w139:bool)  [unwired: 10 in]
            n68 = case shown="True" w139 {
              tunnel: "history length (min)" -> [_ w169]
              tunnel: "save every # (min)" -> [_ w168]
              tunnel: w136 -> [_ w167]
              tunnel: w140 -> [_ w166]
              tunnel: w151 -> [_ w165]
              tunnel: w150 -> [_ w164]
              tunnel: w148 -> [_ w163]
              tunnel: "Sweep folder path" -> [_ w158]
              tunnel: "plot" -> [_ w156]
              tunnel: "plot lever  ?" -> [_ w155]
              frame False {
              }
              frame True {
                n69 = call "capacitor - aggregate.vi"("loss"=w165, "history length (min)"=w169, "save every # (min)"=w168, "aggregate every # sec"=w167, "capacitance"=w166, "time(min)"=w164, "temperature"=w163, "Sweep folder path"=w158) -> ("loss array"=w159:dbl[], "capacitance array"=w162:dbl[], "time(min) array"=w161:dbl[], "temperature array"=w160:dbl[], "delta capacitance array"=w157:dbl[])  [unwired: 3 in]
                n70 = case shown="True" w155 {
                  tunnel: w162 -> [_ w176]
                  tunnel: w161 -> [_ w174]
                  tunnel: w160 -> [_ w173]
                  tunnel: w159 -> [_ w172]
                  tunnel: w157 -> [_ w171]
                  tunnel: w156 -> [_ w170]
                  frame False {
                  }
                  frame True {
                    n71 = case shown="\"Delta Cap vs Temp\"" w170 {
                      tunnel: [w181 w183 w185 w187 w188] -> w177
                      tunnel: w176 -> [w181 w183 _ _ _]
                      tunnel: [w180 w182 w184 w186 w189] -> w175
                      tunnel: w174 -> [w180 _ w184 _ _]
                      tunnel: w173 -> [_ w182 _ w186 w189]
                      tunnel: w172 -> [_ _ w185 w187 _]
                      tunnel: w171 -> [_ _ _ _ w188]
                      frame "Capac vs Time", Default {
                      }
                      frame "Capac vs Temp" {
                      }
                      frame "Loss  vs Time" {
                      }
                      frame "Loss vs Temp" {
                      }
                      frame "Delta Cap vs Temp" {
                      }
                    }
                    n72 = Bundle("temperature array"=w175, "delta capacitance array"=w177) -> (w179:T28)  [unwired: 1 in]
                    n73 = Build Array(w179) -> (→"Plot: capacitance":T29)
                  }
                }
                "Loss" <- w165
                "Capacitance" <- w166
                "time(min)" <- w164
                "temperature" <- w163
              }
            }
            n74 = Build Path(base path="Sweep folder path", name or relative path="ErrorLog.txt") -> (appended path=w144:path)
            n75 = call "BypassAndLogErrors -- V2.vi"("Bypass Errors"=w147, "error in (no error)"=w142, "Log File Path"=w144) -> ("error out"=w141:errorcluster)  [unwired: 8 in]
          }
        }
        n76 = Multiply(x="read AH every # sec", y=1000) -> (x*y=w129:dbl)
        n77 = Wait (ms)(milliseconds to wait=w129) -> ()  [unwired: 1 out]
      }
    }
  }
  n78 = while {
    shift-right: [w193] -> _
    shift-left: "error in" -> [w199]
    tunnel: w10 -> [w209]
    tunnel: w5 -> [w208]
    tunnel: w8 -> [w202]
    tunnel: string[] ["rus loop: on", "rus loop: off", "itc box: off", "itc box: gas zero", "itc box: read state", "itc box: heater auto", "itc box: heater manual and zero", "itc box: set temperature to ([\\d\\.]+)", "itc box: write sweep table", "itc box: read sweep table", "itc box: start/stop sweep", "itc box: set gas to ([\\d\\.]+)", "gas flow: off", "gas flow: on", "gas flow: force up", "gas flow: force down", "gas flow: stop up/down", "gas flow: set gas to \\d+", "gas flow: set gas to", "gas rus itc: stop", "tabs: disable", "tabs: enable", "all: init", "set: new_sweep_table=(.*\\n?)+", "set: new_set_temperature=([\\d\\.]+)"] -> [w197]
    stop <- FALSE stop-if-true
    w195 = TRUE  # Bypass Errors
    w200 = TRUE  # Bypass Errors
    n79 = local read "sweep folder path"() -> (w190:path)
    n80 = local read "temperature indicator panel"() -> (w203:T19)
    n81 = local read "Save data settings"() -> (w196:T8)
    n82 = local read "temperature boxes"() -> (w204:T21)
    n83 = Wait (ms)(milliseconds to wait=u32 11 ("milliseconds per cycle")) -> ()  [unwired: 1 out]
    n84 = control-ref of="Plot: temperature"() -> (w206:refnum<vi>)
    n85 = control-ref of="Plot: heater/gas"() -> (w207:refnum<vi>)
    n86 = call "ctl -- name dispatcher.vi"("sweep folder path"=w190, "ctl name dispatch"=ctl_--_name_dispatcher_--_action."errors" ("ctl kind")) -> ("file path"=w191:path)  [unwired: 7 in, 2 out]
    n87 = call "BypassAndLogErrors -- V2.vi"("Bypass Errors"=w200, "error in (no error)"=w199, "Log File Path"=w191) -> ("error out"=w198:errorcluster)  [unwired: 8 in]
    n88 = event shown="[10] <action>: User Event" {
      selector: w209 -> [_ _ _ _ _ _ _ _ _ _ _ _ _ _ _ _ _ _ _ _]
      dyn-events: _ -> [_ _ _ _ _ _ _ _ _ _ _ _ _ _ _ _ _ _ _ _]
      timeout: 20 -> [_ _ _ _ _ _ _ _ _ _ _ _ _ _ _ _ _ _ _ _]
      tunnel: [_ "upload new sweep table" _ _ _ _ _ _ _ _ _ _ _ _ _ _ _ _ _ _] -> _
      tunnel: w198 -> [w212 w213 w218 w224 w227 w232 w233 w234 w238 w243 w251 w1133 w1142 w1143 w1146 w1149 w1152 w1161 w1162 w1165]
      tunnel: [w212 w213 w218 w224 w227 w232 w233 w234 w238 w243 w247 w1133 w1142 w1143 w1146 w1149 w1152 w1161 w1162 w1165] -> w194
      tunnel: [_ FALSE _ _ _ _ _ _ _ _ _ _ _ _ _ _ _ _ _ _] -> _
      tunnel: [_ _ "Read Sweep Table in the box" _ _ _ _ _ _ _ _ _ _ _ _ _ _ _ _ _] -> _
      tunnel: [_ _ _ _ "set temperature to" "set heater to" _ _ _ _ _ _ _ _ _ _ _ _ _ _] -> _
      tunnel: [_ _ _ _ _ _ _ w237 _ _ _ _ _ _ _ _ _ _ _ _] -> _
      tunnel: TRUE -> [_ _ _ _ _ _ _ _ _ _ _ _ _ _ _ _ _ _ _ _]
      tunnel: w208 -> [_ w214 w220 w223 w226 w231 _ _ w240 w242 w257 _ w1141 w1145 w1147 w1150 w1157 _ w1164 w1167]
      tunnel: w207 -> [_ _ _ _ _ _ _ w236 _ _ _ _ _ _ _ _ _ _ _ _]
      tunnel: w206 -> [_ _ _ _ _ _ _ w235 _ _ _ _ _ _ _ _ _ _ _ _]
      tunnel: w196 -> [_ _ _ _ _ _ _ _ _ _ _ w1138 _ _ _ _ _ _ _ _]
      tunnel: w204 -> [_ _ _ _ _ _ _ _ _ _ w255 w1135 _ _ _ _ _ _ _ _]
      tunnel: w203 -> [_ _ _ _ _ _ _ _ _ _ w254 _ _ _ _ _ _ _ _ _]
      tunnel: w202 -> [_ _ _ _ _ _ _ _ _ _ w253 _ _ _ _ _ _ _ _ _]
      tunnel: w197 -> [_ _ _ _ _ _ _ _ _ _ w250 _ _ _ _ _ _ _ _ _]
      tunnel: w191 -> [_ _ _ _ _ _ _ _ _ _ w244 _ _ _ _ _ _ _ _ _]
      tunnel: w190 -> [_ _ _ _ _ _ _ _ _ _ w246 _ _ _ _ _ _ _ _ _]
      event Timeout {
        n89 = event-data() -> ()  [unwired: 1 in, 2 out]
      }
      event "upload new sweep table": Value Change {
        w215 = "itc box: write sweep table"  # event data
        n90 = event-data() -> ()  [unwired: 1 in, 1 out]
        n91 = Generate User Event(user event=w214, event data cluster=w215) -> ()  [unwired: 2 in, 2 out]
      }
      event "Read Sweep Table in the box": Value Change {
        w219 = "itc box: read sweep table"  # event data
        n92 = event-data() -> ()  [unwired: 1 in, 5 out]
        n93 = Generate User Event(user event=w220, event data cluster=w219) -> ()  [unwired: 2 in, 2 out]
      }
      event Value Change {
        w222 = "itc box: start/stop sweep"  # event data
        n94 = event-data() -> ()  [unwired: 1 in, 1 out]
        n95 = Generate User Event(user event=w223, event data cluster=w222) -> ()  [unwired: 2 in, 2 out]
      }
      event "set temperature to": Value Change {
        n96 = event-data() -> ()  [unwired: 1 in, 5 out]
        n97 = Generate User Event(user event=w226, event data cluster="itc box: set temperature to" ("action")) -> ()  [unwired: 2 in, 2 out]
      }
      event "set heater to": Value Change {
        n98 = event-data() -> ()  [unwired: 1 in, 5 out]
        n99 = Generate User Event(user event=w231, event data cluster="itc box: set heater to" ("action")) -> ()  [unwired: 2 in, 2 out]
      }
      event Key Down {
        n100 = event-data() -> ()  [unwired: 1 in, 2 out]
      }
      event "show plot pallets": Value Change {
        n101 = event-data() -> ("NewVal"=w237:bool)  [unwired: 1 in]
        n102 = property on="Property Node" class="XYGraph (strict)"(reference=w235, "ScaleLegendVis"=w237, "Palette Visible"=w237, "Legend Visible"=w237) -> ()  [unwired: 1 in, 2 out]
        n103 = property on="Property Node" class="XYGraph (strict)"(reference=w236, "ScaleLegendVis"=w237, "Palette Visible"=w237, "Legend Visible"=w237) -> ()  [unwired: 1 in, 2 out]
      }
      event Value Change {
        w239 = "itc box: heater manual and zero"  # event data
        n104 = event-data() -> ()  [unwired: 1 in, 5 out]
        n105 = Generate User Event(user event=w240, event data cluster=w239) -> ()  [unwired: 2 in, 2 out]
      }
      event Value Change {
        w241 = "itc box: heater auto"  # event data
        n106 = event-data() -> ()  [unwired: 1 in, 5 out]
        n107 = Generate User Event(user event=w242, event data cluster=w241) -> ()  [unwired: 2 in, 2 out]
      }
      event User Event {
        n108 = event-data() -> ("action"=w258:string)  [unwired: 1 in]
        n109 = local read "seconds per cycle"() -> (w248:dbl)
        n110 = local read "seconds"() -> (w249:dbl)
        n111 = case shown="\"itc 503 controller: check\"" w258 {
          selector: w258 -> [_ w277 _ w307 _ w327 w333 w339 w344 _ _ _ w381 _ _ _ _ _ _ _ _ _ _ _ _ _ _ _ _ w490 _ w1009 _ _ _ w1026 _ w1041 _ w1069 _ _ _ _ w1088 w1091 w1099]
          tunnel: w249 -> [_ _ w289 _ w311 w323 w328 w334 _ w362 _ _ w376 _ _ _ _ _ _ _ _ _ _ _ _ _ _ _ _ _ _ _ _ _ w1019 w1024 _ _ w1056 _ _ _ _ _ _ _ _]
          tunnel: w257 -> [w262 _ _ _ w317 _ _ _ w341 _ _ _ _ _ _ _ _ w392 _ _ _ _ _ _ _ _ _ _ w470 w485 w992 _ _ _ _ _ _ _ _ _ _ _ _ _ _ _ _]
          tunnel: FALSE -> [_ _ _ _ _ _ _ _ _ _ _ _ _ _ _ _ _ _ _ _ _ _ _ _ _ _ _ _ _ _ _ w1010 w1012 _ _ _ _ _ _ _ _ _ _ _ _ _ _]
          tunnel: w255 -> [_ _ w290 w305 _ _ _ _ _ w361 _ _ w378 _ _ _ _ _ _ _ _ _ w427 _ _ _ _ _ _ _ w994 _ _ _ w1018 _ w1030 _ w1057 _ _ _ _ _ _ _ w1092]
          tunnel: w254 -> [_ _ _ _ _ _ _ _ _ w359 _ _ w377 _ _ _ _ _ _ _ _ _ _ _ _ _ _ _ _ _ _ _ _ _ _ _ _ _ _ _ _ _ _ _ _ _ _]
          tunnel: w253 -> [_ _ _ _ _ _ _ _ w343 _ _ _ _ _ _ _ _ _ _ _ _ _ _ _ _ _ _ _ _ _ _ _ _ _ _ _ _ _ _ _ _ _ _ _ _ _ _]
          tunnel: TRUE -> [_ _ _ _ _ _ _ _ _ _ _ _ _ _ _ _ _ _ _ _ _ _ _ _ _ _ _ _ _ _ _ _ _ w1014 _ _ _ _ _ _ _ _ _ _ _ _ _]
          tunnel: w251 -> [w261 w276 w288 w306 w315 w326 w332 w338 w340 w357 w370 w372 w375 w383 w385 w387 w389 w390 w398 w400 w403 w406 w417 w435 w442 w445 w449 w453 w471 w486 w990 w1008 w1011 w1013 w1017 w1025 w1029 w1043 w1054 w1068 w1072 w1073 w1074 w1079 w1084 w1090 w1098]
          tunnel: [w261 w276 w287 w306 w315 w326 w332 w338 w340 w357 w370 w372 w375 w383 w385 w387 w389 w390 w397 w399 w402 w405 w417 w431 w441 w444 w448 w452 w468 w486 w990 w1008 w1011 w1013 w1017 w1025 w1029 w1042 w1053 w1068 w1072 w1073 w1074 w1079 w1084 w1090 w1097] -> w247
          tunnel: w250 -> [w260 _ _ _ _ _ _ _ _ _ _ _ _ _ _ _ _ _ _ _ _ _ _ _ _ _ _ _ _ _ _ _ _ _ _ _ _ _ _ _ _ _ _ _ _ _ _]
          tunnel: w248 -> [_ _ _ _ _ _ _ _ _ _ _ _ _ _ _ _ _ _ _ _ _ _ _ _ _ _ _ _ _ _ _ _ _ _ _ _ _ _ w1055 _ _ _ _ _ _ _ w1095]
          tunnel: w246 -> [_ _ w282 _ _ _ _ _ _ _ _ _ _ _ _ _ _ _ _ _ _ _ _ _ _ _ _ _ _ _ _ _ _ _ w1015 _ w1028 w1039 _ _ _ _ _ _ _ _ w1096]
          tunnel: "disable interaction with itc" -> [_ _ _ _ _ _ _ _ _ _ _ _ _ _ _ _ _ _ _ _ _ _ _ _ _ _ _ _ _ _ _ _ _ _ _ _ _ w1037 w1052 _ _ _ _ _ _ _ _]
          tunnel: w244 -> [_ _ _ _ _ _ _ _ _ _ _ _ _ _ _ _ _ _ _ _ _ _ _ _ _ _ _ _ _ _ _ _ _ _ _ _ _ _ w1051 _ _ _ _ _ _ _ _]
          frame "9ctl: check" {
            # "list of commands understood by protocol"
            n112 = call "p9ctl.vi"("p9 action"=p9action_control."check") -> ("ctl"=w264:string, "news?"=w263:bool)  [unwired: 8 in, 1 out]
            n113 = case shown="True" w263 {
              tunnel: w264 -> [_ w266]
              tunnel: w262 -> [_ w267]
              tunnel: w260 -> [_ w270]
              frame False {
              }
              frame True {
                n114 = call "test for a regexp list.vi"("quote specials"=FALSE, "string"=w266, "regexps"=w270) -> ("whole match"=w265:string, "match found"=w268:bool)  [unwired: 5 in, 2 out]
                n115 = case shown="True" w268 {
                  tunnel: w267 -> [_ w272]
                  tunnel: w265 -> [_ w271]
                  frame False {
                  }
                  frame True {
                    n116 = Generate User Event(user event=w272, event data cluster=w271) -> ()  [unwired: 2 in, 2 out]
                  }
                }
              }
            }
          }
          frame "9ctl: init" {
            w273 = path "C:/Users/riggslab/Dropbox/ultrasound_experiment/9ctl"  # ctl path
            n117 = call "sweep init checklist.vi"("action"=w277) -> ()  [unwired: 10 in, 1 out]
            n118 = call "p9ctl.vi"("p9 action"=p9action_control."init", "ctl path"=w273) -> ("9ctl OK"=→"9ctl OK":bool)  [unwired: 7 in, 2 out]
          }
          frame "PID: check" {
            n119 = Unbundle By Name(w290) -> ("ITC temperature"=w281:dbl)
            n120 = control-ref of="PID timer"() -> (w285:refnum<vi>)
            n121 = call "slider timer .vi"("interval (sec)"=100.0, "action"=countdown_control."check", "timer ref"=w285) -> ("tic"=w284:bool)  [unwired: 6 in, 2 out]
            n122 = call "Q -- check range -- i -- real.vi"("lower"=0.01, "number"=w281) -> ("in range?"=w279:bool)  [unwired: 7 in, 2 out]
            n123 = And(x=w279, y=w284) -> (x .and. y?=w283:bool)
            n124 = case shown="True" w283 {
              tunnel: w289 -> [_ _]
              tunnel: w281 -> [_ w298]
              tunnel: w288 -> [w291 w297]
              tunnel: [w291 w296] -> w287
              tunnel: w282 -> [_ w294]
              frame False {
              }
              frame True {
                w295 = enum16{"CHECK", "INIT"}."CHECK"  # action
                n125 = call "Control PID - V1.vi"("action"=w295, "ITC temperature"=w298, "error in"=w297, "sweep folder path"=w294) -> ("error out"=w296:errorcluster, "PID"=→"PID":dbl[], "OK?"=→"PID OK":bool)  [unwired: 5 in]
                "PID temperature" <- w298
              }
            }
          }
          frame "PID: init" {
            w299 = countdown_control."start" ("action")
            w304 = enum16{"CHECK", "INIT"}."INIT"  # action
            n126 = Unbundle By Name(w305) -> ("ITC temperature"=w303:dbl)
            n127 = call "sweep init checklist.vi"("action"=w307) -> ()  [unwired: 10 in, 1 out]
            n128 = control-ref of="PID timer"() -> (w302:refnum<vi>)
            n129 = call "slider timer .vi"("interval (sec)"=100.0, "action"=w299, "timer ref"=w302) -> ("timer out"=w300:refnum<vi>)  [unwired: 6 in, 2 out]
            n130 = call "slider timer .vi"("action"=w299, "timer ref"=w300) -> ()  [unwired: 7 in, 3 out]
            n131 = call "Control PID - V1.vi"("action"=w304, "ITC temperature"=w303) -> ()  [unwired: 7 in, 3 out]
          }
          frame "alarm clock: check" {
            w314 = enum16{"init", "check", "start", "stop"}."check"  # action
            n132 = call "alarm clock - fancy.vi"("action"=w314, "alarm"="alarm", "seconds"=w311) -> ("alarm out"=w312:T20, "alarm!"=w310:bool)  [unwired: 7 in]
            n133 = And(x=w310, y=FALSE) -> (x .and. y?=w308:bool)
            n134 = case shown="True" w308 {
              tunnel: w317 -> [_ w319]
              tunnel: string[] ["gas flow: off", "rus loop: off", "itc box: off"] -> [_ w318]
              frame False {
              }
              frame True {
                n135 = for {
                  tunnel: w319 -> [w321]
                  tunnel: w318 -> [w320] mode=indexing
                  n136 = Generate User Event(user event=w321, event data cluster=w320) -> ()  [unwired: 2 in, 2 out]
                }
              }
            }
            n137 = local write "alarm"(w312) -> ()
          }
          frame "alarm clock: init" {
            w322 = enum16{"init", "check", "start", "stop"}."init"  # action
            n138 = local read "alarm"() -> (w325:T20)
            n139 = call "sweep init checklist.vi"("action"=w327) -> ()  [unwired: 10 in, 1 out]
            n140 = call "alarm clock - fancy.vi"("action"=w322, "alarm"=w325, "seconds"=w323) -> ("alarm out"=w324:T20)  [unwired: 7 in, 1 out]
            n141 = local write "alarm"(w324) -> ()
          }
          frame "alarm clock: start" {
            w331 = enum16{"init", "check", "start", "stop"}."start"  # action
            n142 = local read "alarm"() -> (w330:T20)
            n143 = call "sweep init checklist.vi"("action"=w333) -> ()  [unwired: 10 in, 1 out]
            n144 = call "alarm clock - fancy.vi"("action"=w331, "alarm"=w330, "seconds"=w328) -> ("alarm out"=w329:T20)  [unwired: 7 in, 1 out]
            n145 = local write "alarm"(w329) -> ()
          }
          frame "alarm clock: stop" {
            w337 = enum16{"init", "check", "start", "stop"}."stop"  # action
            n146 = local read "alarm"() -> (w336:T20)
            n147 = call "sweep init checklist.vi"("action"=w339) -> ()  [unwired: 10 in, 1 out]
            n148 = call "alarm clock - fancy.vi"("action"=w337, "alarm"=w336, "seconds"=w334) -> ("alarm out"=w335:T20)  [unwired: 7 in, 1 out]
            n149 = local write "alarm"(w335) -> ()
          }
          frame "all: init" {
            n150 = for {
              tunnel: w343 -> [w347] mode=indexing
              tunnel: [w345] -> w342 mode=indexing
              n151 = Concatenate Strings(w347, " init" ("event data")) -> (w345:string)
            }
            n152 = call "sweep init checklist.vi"("list"=w342, "init str"=w344, "action"=w344) -> ()  [unwired: 8 in, 1 out]
            n153 = for {
              tunnel: w341 -> [w349]
              tunnel: w342 -> [w348] mode=indexing
              n154 = Generate User Event(user event=w349, event data cluster=w348) -> ()  [unwired: 2 in, 2 out]
            }
          }
          frame "gas flow: check" {
            n155 = Unbundle By Name(w359) -> ("heater i-average, V"=w358:dbl)
            n156 = Unbundle By Name(w361) -> ("gas flow"=w360:dbl)  [unwired: 1 out]
            n157 = call "gas flow controller- V2.vi"("gas flow, %"=w360, "action"=gas_flow_controller_action."check", "heater"=w358, "seconds"=w362) -> ("gas flow controller out"=w356:T17)  [unwired: 7 in]
            n158 = Unbundle By Name(w356) -> ("ramp Up progress"=→"ramp Up progress":T18, "ramp Down progress"=→"ramp Down progress":T18, "state"=w352:enum16{"normal", "ramp up", "ramp down"})
            n159 = case shown="\"ramp down\"" w352 {
              tunnel: [FALSE TRUE FALSE] -> w351
              tunnel: [TRUE FALSE FALSE] -> w350
              frame "ramp up" {
              }
              frame "ramp down" {
              }
              frame "normal", Default {
              }
            }
            n160 = property on="ramp Up progress" class="Clust (strict)"("Visible"=w350) -> ()  [unwired: 2 in, 2 out]
            n161 = property on="ramp Down progress" class="Clust (strict)"("Visible"=w351) -> ()  [unwired: 2 in, 2 out]
          }
          frame "gas flow: force down" {
            n162 = call "gas flow controller- V2.vi"("action"=gas_flow_controller_action."force DOWN") -> ()  [unwired: 10 in, 1 out]
          }
          frame "gas flow: force up" {
            n163 = call "gas flow controller- V2.vi"("action"=gas_flow_controller_action."force UP") -> ()  [unwired: 10 in, 1 out]
          }
          frame "gas flow: init" {
            n164 = Unbundle By Name(w378) -> ("heater"=w379:dbl, "gas flow"=w380:dbl)
            n165 = Unbundle By Name(w377) -> ()  [unwired: 1 out]
            n166 = call "sweep init checklist.vi"("action"=w381) -> ()  [unwired: 10 in, 1 out]
            n167 = control-ref of="gas flow controller"() -> (w373:refnum<vi>)
            n168 = call "gas flow controller- V2.vi"("gas flow, %"=w380, "action"=gas_flow_controller_action."init", "heater"=w379, "gas flow controller ref"=w373, "seconds"=w376) -> ()  [unwired: 6 in, 1 out]
          }
          frame "gas flow: off" {
            n169 = call "gas flow controller- V2.vi"("action"=gas_flow_controller_action."turn off") -> ()  [unwired: 10 in, 1 out]
          }
          frame "gas flow: on" {
            n170 = call "gas flow controller- V2.vi"("action"=gas_flow_controller_action."turn on") -> ()  [unwired: 10 in, 1 out]
          }
          frame "gas flow: set gas to" {
            n171 = call "gas flow controller- V2.vi"("action"=gas_flow_controller_action."set gas to") -> ()  [unwired: 10 in, 1 out]
          }
          frame "gas flow: stop up/down" {
            n172 = call "gas flow controller- V2.vi"("action"=gas_flow_controller_action."stop UP/DOWN") -> ()  [unwired: 10 in, 1 out]
          }
          frame "gas rus itc: stop" {
            n173 = for {
              tunnel: w392 -> [w394]
              tunnel: string[] ["gas flow: off", "rus loop: off", "itc box: off"] -> [w393] mode=indexing
              n174 = Generate User Event(user event=w394, event data cluster=w393) -> ()  [unwired: 2 in, 2 out]
            }
          }
          frame "itc box: gas zero" {
            w395 = itc_503_box_-_control."set gas to"  # itc box action
            w396 = 1.0  # Gas %
            n175 = call "itc Hg box controller.vi"("itc box action"=w395, "error in"=w398, "input"=w396) -> ("error out"=w397:errorcluster)  [unwired: 6 in, 2 out]
          }
          frame "itc box: heater auto" {
            w401 = itc_503_box_-_control."heater auto"  # itc box action
            n176 = call "itc Hg box controller.vi"("itc box action"=w401, "error in"=w400) -> ("error out"=w399:errorcluster)  [unwired: 7 in, 2 out]
          }
          frame "itc box: heater manual and zero" {
            w404 = itc_503_box_-_control."heater manual and zero"  # itc box action
            n177 = call "itc Hg box controller.vi"("itc box action"=w404, "error in"=w403) -> ("error out"=w402:errorcluster)  [unwired: 7 in, 2 out]
          }
          frame "itc box: off" {
            w407 = itc_503_box_-_control."shut off"  # itc box action
            n178 = call "itc Hg box controller.vi"("itc box action"=w407, "error in"=w406) -> ("error out"=w405:errorcluster)  [unwired: 7 in, 2 out]
          }
          frame "itc box: read state" {
            (unwired) "\nsweeptable=\n"
            n179 = local read "date string Array"() -> (w410:string[])
            n180 = local read "Sweep Table"() -> (w411:dbl[][])
            n181 = Unbundle By Name(w427) -> ("ITC temperature"=w426:dbl, "ITC set temperature"=w409:dbl, "LTC temperature"=w425:dbl, "heater"=w424:dbl, "gas flow"=w423:dbl, "P"=w422:dbl, "D"=w421:dbl, "I"=w420:dbl, "ITC state"=w419:string, "nonzero temperature"=w413:dbl)
            n182 = call "string -- format sweep table string.vi"("ITC set temperature"=w409, "date string Array"=w410, "Sweep Table"=w411) -> ("string out"=w408:string)  [unwired: 8 in]
            n183 = Format Into String(format string="itc=%4f  itc_set=%4f  ltc=%4f  heater=%3f  gas=%3f  P=%3f  D=%3f  I=%3f  itc_state=%s  nzt=%3f" ("action"), w426, w409, w425, w424, w423, w422, w421, w420, w419, w413) -> (resulting string=w416:string)  [unwired: 2 in, 1 out]
            n184 = Concatenate Strings(w416, "\r", w408) -> (w415:string)
            n185 = call "p9ctl.vi"("p9 action"=p9action_control."message", "message"=w415) -> ()  [unwired: 7 in, 3 out]
          }
          frame "itc box: read sweep table" {
            w437 = T34."table to rates"  # action
            # "read sweep table"
            n186 = call "itc Hg box controller.vi"("itc box action"=itc_503_box_-_control."read sweep table", "error in"=w435) -> ("error out"=w432:errorcluster, "Sweep Table"=w434:dbl[][])  [unwired: 7 in, 1 out]
            "Sweep Table" <- w434
            n187 = call "itc Hg box controller.vi"("itc box action"=itc_503_box_-_control."read state", "error in"=w432) -> ("error out"=w431:errorcluster, "itc box state OUT"=w429:T38)  [unwired: 7 in, 1 out]
            n188 = Unbundle By Name(w429) -> ("ITC set temperature"=w428:dbl)
            "current set temperature" <- w428
            n189 = call "sweep table staff.vi"("action"=w437, "Sweep Table"=w434, "set temperature IN"=w428) -> ("date string Array"=→"date string Array":string[], "Sweep Rates , min/K"=→"Sweep Rates , min/K":dbl[])  [unwired: 5 in, 2 out]
          }
          frame "itc box: set gas to" {
            n190 = call "itc Hg box controller.vi"("itc box action"=itc_503_box_-_control."set gas to", "error in"=w442, "input"="set gas % to") -> ("error out"=w441:errorcluster)  [unwired: 6 in, 2 out]
          }
          frame "itc box: set temperature to" {
            n191 = call "itc Hg box controller.vi"("itc box action"=itc_503_box_-_control."set temperature to", "error in"=w445, "input"="itc box: set temperature to: value") -> ("error out"=w444:errorcluster)  [unwired: 6 in, 2 out]
          }
          frame "itc box: set heater to" {
            n192 = call "itc Hg box controller.vi"("itc box action"=itc_503_box_-_control."set heater to", "error in"=w449, "input"="itc box: set heater to: value") -> ("error out"=w448:errorcluster)  [unwired: 6 in, 2 out]
          }
          frame "itc box: start/stop sweep" {
            n193 = local read "ITC panel"() -> (w454:T15)
            n194 = Unbundle By Name(w454) -> ("in sweep"=w455:bool)
            n195 = case shown="True" w455 {
              tunnel: [itc_503_box_-_control."start sweep" ("itc box action") itc_503_box_-_control."stop sweep" ("itc box action")] -> w451
              frame False {
                # "start sweep ..."
              }
              frame True {
                # "stop sweep ..."
              }
            }
            n196 = call "itc Hg box controller.vi"("itc box action"=w451, "error in"=w453) -> ("error out"=w452:errorcluster)  [unwired: 7 in, 2 out]
          }
          frame "itc box: write sweep table" {
            w458 = TRUE
            w472 = FALSE
            n197 = local write "Uploading ..."(w458) -> ()
            n198 = property on="Uploading ..." class="Bool (strict)"(error in=w471, "Visible"=w458) -> (error out=w463:errorcluster)  [unwired: 1 in, 1 out]
            n199 = case shown="True" "use" {
              tunnel: [w474 w479] -> w461
              tunnel: "new sweep table" -> [w474 w482]
              tunnel: "Rates , min/K" -> [w476 w483]
              tunnel: "set temperature" -> [w475 w484]
              frame False {
                n200 = call "sweep table staff.vi"("action"=T34."table to rates", "Sweep Table"=w474, "Sweep Rates , min/K IN"=w476, "set temperature IN"=w475) -> ("Sweep Rates , min/K"=w473:dbl[])  [unwired: 4 in, 3 out]
                n201 = local write "Rates , min/K"(w473) -> ()
              }
              frame True {
                n202 = call "sweep table staff.vi"("action"=T34."rates to table", "Sweep Table"=w482, "Sweep Rates , min/K IN"=w483, "set temperature IN"=w484) -> ("date string Array"=w478:string[], "Sweep Table"=w479:dbl[][], "Sweep Rates , min/K"=w480:dbl[])  [unwired: 4 in, 1 out]
                n203 = local write "new sweep table"(w479) -> ()
                n204 = local write "date string Array"(w478) -> ()
                n205 = local write "Sweep Rates , min/K"(w480) -> ()
              }
            }
            n206 = call "itc Hg box controller.vi"("itc box action"=itc_503_box_-_control."write sweep table", "error in"=w463, "Sweep Table In"=w461, "input"="set temperature") -> ("error out"=w459:errorcluster)  [unwired: 5 in, 2 out]
            n207 = local write "Uploading ..."(w472) -> ()
            n208 = property on="Uploading ..." class="Bool (strict)"(error in=w459, "Visible"=w472) -> (error out=w469:errorcluster)  [unwired: 1 in, 1 out]
            n209 = Generate User Event(user event=w470, event data cluster="itc box: read sweep table", error in=w469) -> (error out=w468:errorcluster)  [unwired: 1 in, 1 out]
          }
          frame "nothing", Default {
            w492 = FALSE  # quote specials
            # "intercept actions that do not match anything on the list"
            n210 = call "test for a regexp list.vi"("quote specials"=w492, "string"=w490, "regexps"=string[] ["itc\\ box:\\ set\\ gas\\ to\\ ([\\d\\.]+)", "itc\\ box:\\ set\\ temperature\\ to\\ ([\\d\\.]+)", "set:\\ new_sweep_table=(\\s*\\n)?((.*\\n?)+)", "set:\\ new_set_temperature=([\\d\\.]+)"]) -> ("match found"=w491:bool, "matching string index"=w487:i32, "matching regexp"=w489:string)  [unwired: 5 in, 1 out]
            n211 = case shown="True" w491 {
              tunnel: w490 -> [_ w496]
              tunnel: w489 -> [_ w494]
              tunnel: w487 -> [_ w495]
              tunnel: w485 -> [_ w493]
              frame False {
              }
              frame True {
                n212 = case shown="1" w495 {
                  tunnel: w496 -> [_ w500 w625 w754 w875]
                  tunnel: w494 -> [_ w499 w624 w755 w876]
                  tunnel: w493 -> [_ w498 w623 _ _]
                  frame -1, Default {
                  }
                  frame 1 {
                    n213 = xnode "Match Regular Expression"("input string"=w500, "regular expression"=w499) -> ("submatch 1"=w501:string)  [unwired: 4 in, 5 out]
                    n214 = flat-sequence {
                      tunnel: w501 -> [w506]
                      tunnel: w498 -> [w508]
                      tunnel: "itc box: set temperature to" ("action") -> [w507]
                      frame #0 {
                        w503 = 1.0  # lower
                        w504 = 330.0  # upper
                        n215 = Fract/Exp String To Number(string=w506) -> (number=w505:dbl)  [unwired: 3 in, 1 out]
                        n216 = call "Q -- check range.vi"("upper"=w504, "lower"=w503, "number"=w505) -> ("number in range"=w502:dbl)  [unwired: 4 in, 4 out]
                        n217 = local write "itc box: set temperature to: value"(w502) -> ()
                      }
                      frame #1 {
                        n218 = Generate User Event(user event=w508, event data cluster=w507) -> ()  [unwired: 2 in, 2 out]
                      }
                    }
                  }
                  frame 0 {
                    n219 = xnode "Match Regular Expression"("input string"=w625, "regular expression"=w624) -> ("submatch 1"=w626:string)  [unwired: 4 in, 5 out]
                    n220 = flat-sequence {
                      tunnel: w626 -> [w631]
                      tunnel: w623 -> [w633]
                      tunnel: "itc box: set gas to" ("action") -> [w632]
                      frame #0 {
                        w629 = 0.1  # lower
                        w630 = 99.0  # upper
                        n221 = Fract/Exp String To Number(string=w631) -> (number=w628:dbl)  [unwired: 3 in, 1 out]
                        n222 = call "Q -- check range.vi"("upper"=w630, "lower"=w629, "number"=w628) -> ("number in range"=w627:dbl)  [unwired: 4 in, 4 out]
                        n223 = local write "set gas % to"(w627) -> ()
                      }
                      frame #1 {
                        n224 = Generate User Event(user event=w633, event data cluster=w632) -> ()  [unwired: 2 in, 2 out]
                      }
                    }
                  }
                  frame 2 {
                    w748 = 0
                    (unwired) "\t"
                    n225 = local read "new sweep table"() -> (w750:dbl[][])
                    n226 = xnode "Match Regular Expression"("input string"=w754, "regular expression"=w755) -> ("submatch 2"=w752:string)  [unwired: 4 in, 6 out]
                    n227 = Spreadsheet String To Array(delimiter (Tab)=string[] [" ", "\t"], format string="%f " ("delimiter (Tab)"), spreadsheet string=w752) -> (array=w749:dbl[][])  [unwired: 1 in]
                    n228 = Replace Array Subset(array=w750, new element=w749, index (row)=w748, index (col)=w748) -> (w747:dbl[][])
                    n229 = local write "new sweep table"(w747) -> ()
                  }
                  frame 3 {
                    w871 = 330.0  # upper
                    w872 = 0.0  # lower
                    (unwired) "\t"
                    n230 = xnode "Match Regular Expression"("input string"=w875, "regular expression"=w876) -> ("submatch 1"=w874:string)  [unwired: 4 in, 5 out]
                    n231 = Fract/Exp String To Number(string=w874) -> (number=w873:dbl)  [unwired: 3 in, 1 out]
                    n232 = call "Q -- check range.vi"("upper"=w871, "lower"=w872, "number"=w873) -> ("number in range"=w870:dbl)  [unwired: 4 in, 4 out]
                    n233 = local write "set temperature"(w870) -> ()
                  }
                }
              }
            }
          }
          frame "overheat: check" {
            n234 = Unbundle By Name(w994) -> ("nonzero temperature"=w993:dbl)
            n235 = Not(x="Overheat !!") -> (.not. x?=w998:bool)
            n236 = Greater Or Equal?(x=w993, y="Over heat Temperature") -> (x >= y?=w997:bool)
            n237 = Compound Arithmetic op=AND("Overheat protection", w998, w997) -> (w996:bool)
            n238 = case shown="True" w996 {
              tunnel: [FALSE ("Boolean") TRUE ("Boolean")] -> w1001
              tunnel: w992 -> [_ w1003]
              tunnel: string[] ["gas flow: off", "rus loop: off", "itc box: off", "tabs: disable"] -> [_ w1004]
              frame False {
                (unwired) TRUE ("Control Gas flow ?")
              }
              frame True {
                n239 = for {
                  tunnel: w1003 -> [w1007]
                  tunnel: w1004 -> [w1006] mode=indexing
                  n240 = Generate User Event(user event=w1007, event data cluster=w1006) -> ()  [unwired: 2 in, 2 out]
                }
              }
            }
            n241 = local write "Overheat !!"(w1001) -> ()
          }
          frame "overheat: init" {
            n242 = call "sweep init checklist.vi"("action"=w1009) -> ()  [unwired: 10 in, 1 out]
            n243 = local write "Overheat protection"(w1010) -> ()
            n244 = local write "Overheat !!"(w1010) -> ()
          }
          frame "rus loop: off" {
            n245 = local write "RUS loop"(w1012) -> ()
          }
          frame "rus loop: on" {
            n246 = local write "RUS loop"(w1014) -> ()
          }
          frame "save log: check" {
            n247 = local read "save log"() -> (w1020:T23)
            n248 = call "save ITC log.vi"("action"=enum16{"init", "check"}."check", "file path"=w1015, "temperature boxes"=w1018, "seconds"=w1019, "save log"=w1020) -> ("saving log to"=w1022:string, "save log out"=w1021:T23)  [unwired: 5 in]
            n249 = local write "saving log to"(w1022) -> ()
            n250 = local write "save log"(w1021) -> ()
          }
          frame "save log: init" {
            n251 = call "sweep init checklist.vi"("action"=w1026) -> ()  [unwired: 10 in, 1 out]
            n252 = call "save ITC log.vi"("action"=enum16{"init", "check"}."init", "seconds"=w1024) -> ()  [unwired: 8 in, 2 out]
          }
          frame "stability log: write" {
            n253 = case shown="True" FALSE {
              tunnel: w1030 -> [_ w1033]
              tunnel: w1028 -> [_ w1032]
              frame False {
              }
              frame True {
                (unwired) "Stability_" ("current sweep file name")
                n254 = local read "file name prefix"() -> (w1031:string)
                n255 = call "RUS Sweep -- write line to log file.vi"("temperature boxes"=w1033, "base path"=w1032, "current sweep file name"=w1031, "base name"="Stability_") -> ("writing to"=→"writing log to":string, "log line"=→"log line":string)  [unwired: 5 in, 1 out]
              }
            }
          }
          frame "itc 503 controller: init" {
            n256 = call "sweep init checklist.vi"("action"=w1041) -> ()  [unwired: 10 in, 1 out]
            n257 = call "ctl -- name dispatcher.vi"("sweep folder path"=w1039, "ctl name dispatch"=ctl_--_name_dispatcher_--_action."errors" ("ctl kind")) -> ("file path"=w1038:path)  [unwired: 7 in, 2 out]
            n258 = case shown="\"use oxford ITC\", Default" w1037 {
              tunnel: [itc_503_box_-_control."enable" ("itc box action") itc_503_box_-_control."disable" ("itc box action")] -> w1045
              frame "use oxford ITC", Default {
              }
              frame "do not use oxford ITC" {
              }
            }
            n259 = Unbundle By Name("temperature boxes") -> ("ITC503 Address"=w1048:refnum<visa-resource-name>)
            n260 = call "itc Hg box controller.vi"("itc box action"=w1045, "error in"=w1043) -> ("error out"=w1047:errorcluster)  [unwired: 7 in, 2 out]
            n261 = call "itc Hg box controller.vi"("Log File Path"=w1038, "itc box action"=itc_503_box_-_control."init", "error in"=w1047, "VISA resource name"=w1048) -> ("error out"=w1042:errorcluster)  [unwired: 5 in, 2 out]
          }
          frame "itc 503 controller: check" {
            (unwired) u32 1  # plot every # sec
            w1063 = 60.0  # plot last (min)
            (unwired) u32 1  # aggregate every # sec
            w1062 = 10.0  # history length (min)
            n262 = control-ref of="ITC panel"() -> (w1060:refnum<vi>)
            n263 = call "ITC503 -- scan ITC LTC state.vi"("error logfile path"=w1051, "disable interaction with itc"=w1052, "error in"=w1054, "state IN"=w1057) -> ("error out"=w1053:errorcluster, "itc box state OUT"=w1067:T38, "state OUT"=w1066:T21)  [unwired: 5 in]
            n264 = call "itc ltc - aggregate.vi"("aggregate every # sec"=w1055, "history length (min)"=w1062, "temperature boxes"=w1066) -> ("temperature indicator panel"=w1061:T19)  [unwired: 8 in]
            n265 = call "ITC panel control.vi"("itc box state"=w1067, "action"=T35."parse", "ITC panel IN"=w1060) -> ()  [unwired: 8 in, 1 out]
            n266 = control-ref of="Plot: temperature"() -> (w1058:refnum<vi>)
            n267 = control-ref of="Plot: heater/gas"() -> (w1059:refnum<vi>)
            n268 = local write "temperature boxes"(w1066) -> ()
            n269 = local write "temperature indicator panel"(w1061) -> ()
            n270 = call "itc ltc plots.vi"("Plot: heater/gas"=w1059, "aggregate every # sec"=w1055, "Plot: temperature"=w1058, "plot length (min)"=w1063, "plot?"="plot?", "temperature indicator panel"=w1061, "time (sec)"=w1056) -> ()  [unwired: 5 in]
          }
          frame "sweep table: init" {
            w1071 = FALSE
            n271 = property on="Uploading ..." class="Bool (strict)"("Visible"=w1071) -> ()  [unwired: 2 in, 2 out]
            n272 = call "sweep init checklist.vi"("action"=w1069) -> ()  [unwired: 10 in, 1 out]
            "Uploading ..." <- w1071
            "saving sweep table to" <- "" ("saving sweep table to")
          }
          frame "sweep table: check" {
          }
          frame "tabs: check" {
          }
          frame "tabs: disable" {
            n273 = Select(t=T36."Disabled and Grayed Out" ("Disabled"), s=TRUE, f=T36."Enabled" ("Disabled")) -> (s? t:f=w1076:T36)
            n274 = property on="Tab: ITC controls" class="TabCtl (strict)"("DisabledEnum"=w1076) -> ()  [unwired: 2 in, 2 out]
          }
          frame "tabs: enable" {
            n275 = Select(t=T36."Disabled and Grayed Out" ("Disabled"), s=FALSE, f=T36."Enabled" ("Disabled")) -> (s? t:f=w1081:T36)
            n276 = property on="Tab: ITC controls" class="TabCtl (strict)"("DisabledEnum"=w1081) -> ()  [unwired: 2 in, 2 out]
          }
          frame "tabs: init" {
            n277 = call "sweep init checklist.vi"("action"=w1088) -> ()  [unwired: 10 in, 1 out]
            n278 = Select(t=T36."Disabled and Grayed Out" ("Disabled"), s=FALSE, f=T36."Enabled" ("Disabled")) -> (s? t:f=w1085:T36)
            n279 = property on="Tab: ITC controls" class="TabCtl (strict)"("DisabledEnum"=w1085) -> ()  [unwired: 2 in, 2 out]
          }
          frame "set temperature loop: init" {
            n280 = call "sweep init checklist.vi"("action"=w1091) -> ()  [unwired: 10 in, 1 out]
          }
          frame "set temperature loop: check" {
            n281 = call "sweep init checklist.vi"("action"=w1099) -> ()  [unwired: 10 in, 1 out]
            n282 = Unbundle By Name("Set Temperature PID") -> ("set temperature?"=w1094:bool)
            n283 = case shown="True" w1094 {
              tunnel: w1096 -> [_ w1117]
              tunnel: w1098 -> [w1100 w1115]
              tunnel: [w1100 w1114] -> w1097
              tunnel: w1095 -> [_ w1111]
              tunnel: "Set Temperature PID" -> [_ w1113]
              tunnel: w1092 -> [_ w1103]
              frame False {
              }
              frame True {
                n284 = Bundle By Name(cluster=w1113, "interval(sec)"=w1111) -> (w1112:T14)
                n285 = Unbundle By Name(w1103) -> ("LTC21 Address"=w1102:refnum<visa-resource-name>, "Neocera sensor"=w1101:i32)
                n286 = call "set temperature SINEWAVE - V1.vi"("sweep folder path"=w1117, "Set Temperature PID"=w1112) -> ("next set temperature"=w1116:dbl, "Set Temperature PID OUT"=w1105:T14)  [unwired: 6 in, 2 out]
                n287 = Unbundle By Name(w1105) -> ("Time(min)"=w1109:dbl, "Temperature(K)"=w1108:dbl, "OK?"=w1107:bool, "interval(sec)"=w1106:dbl)
                n288 = case shown="\"set T -> ITC (oxford)\", Default" "set  T target" {
                  tunnel: w1116 -> [w1124 w1128]
                  tunnel: w1115 -> [w1121 w1126]
                  tunnel: [w1120 w1125] -> w1114
                  tunnel: w1102 -> [w1123 _]
                  tunnel: w1101 -> [w1118 _]
                  frame "set T -> LTC (neocera)" {
                    n289 = call "Neocera21 Set T -V1.vi"("Channel"=w1118, "Ramp rate, K/min"=0.03, "error in (no error)"=w1121, "Approach"=Neocera_Set_Point_Aproach."Instant", "Set T"=w1124, "VISA Resource Name"=w1123) -> ("error out"=w1120:errorcluster)  [unwired: 4 in, 1 out]
                  }
                  frame "set T -> ITC (oxford)", Default {
                    n290 = call "itc Hg box controller.vi"("itc box action"=itc_503_box_-_control."set temperature to", "error in"=w1126, "input"=w1128) -> ("error out"=w1125:errorcluster)  [unwired: 6 in, 2 out]
                  }
                }
                n291 = Bundle By Name(cluster=w1105, "Time(min)"=w1109, "Temperature(K)"=w1108, "OK?"=w1107, "interval(sec)"=w1106) -> (w1110:T14)
                n292 = local write "Set Temperature PID"(w1110) -> ()
              }
            }
          }
        }
      }
      event Value Change {
        n293 = event-data() -> ()  [unwired: 1 in, 2 out]
        n294 = Unbundle By Name(w1135) -> ("nonzero temperature"=w1134:dbl)
        n295 = local read "Fast sweep settings"() -> (w1132:T7)
        n296 = call "file name prefix.vi"("Fast sweep settings"=w1132, "temperature"=w1134) -> ("minutes/sweep"=w1131:dbl, "kHz/second"=w1139:dbl, "file name prefix"=w1137:string)  [unwired: 6 in, 1 out]
        n297 = local write "sweep time  (min)"(w1131) -> ()
        n298 = Bundle By Name(cluster=w1138, "File Prefix"=w1137) -> (w1136:T8)
        n299 = Multiply(x=60.0, y=w1131) -> (x*y=→"sweep time (sec)":dbl)
        n300 = local write "kHz/second"(w1139) -> ()
        n301 = local write "Save data settings"(w1136) -> ()
      }
      event Value Change {
        w1140 = "gas flow: set gas to"  # event data
        n302 = event-data() -> ()  [unwired: 1 in, 1 out]
        n303 = Generate User Event(user event=w1141, event data cluster=w1140) -> ()  [unwired: 2 in, 2 out]
      }
      event Value Change {
        w1144 = "gas flow: force up"  # event data
        n304 = event-data() -> ()  [unwired: 1 in, 1 out]
        n305 = Generate User Event(user event=w1145, event data cluster=w1144) -> ()  [unwired: 2 in, 2 out]
      }
      event Value Change {
        w1148 = "gas flow: force down"  # event data
        n306 = event-data() -> ()  [unwired: 1 in, 1 out]
        n307 = Generate User Event(user event=w1147, event data cluster=w1148) -> ()  [unwired: 2 in, 2 out]
      }
      event Value Change {
        w1151 = "gas flow: stop up/down"  # event data
        n308 = event-data() -> ()  [unwired: 1 in, 1 out]
        n309 = Generate User Event(user event=w1150, event data cluster=w1151) -> ()  [unwired: 2 in, 2 out]
      }
      event Value Change {
        w1158 = T39."turn on"  # action
        w1159 = T39."turn off"  # action
        n310 = event-data() -> ("NewVal"=w1156:bool)  [unwired: 1 in]
        n311 = Select(t=w1158, s=w1156, f=w1159) -> ()  [unwired: 1 out]
        n312 = Select(t="gas flow: on" ("event data"), s=w1156, f="gas flow: off" ("event data")) -> (s? t:f=w1153:string)
        n313 = Generate User Event(user event=w1157, event data cluster=w1153) -> ()  [unwired: 2 in, 2 out]
      }
      event Value Change {
        n314 = event-data() -> ()  [unwired: 1 in, 1 out]
        n315 = call "gas flow controller- V2.vi"("action"=gas_flow_controller_action."update parameters") -> ()  [unwired: 10 in, 1 out]
      }
      event Value Change {
        w1163 = "alarm clock: start"  # event data
        n316 = event-data() -> ()  [unwired: 1 in, 2 out]
        n317 = Generate User Event(user event=w1164, event data cluster=w1163) -> ()  [unwired: 2 in, 2 out]
      }
      event Value Change {
        w1166 = "alarm clock: stop"  # event data
        n318 = event-data() -> ()  [unwired: 1 in, 2 out]
        n319 = Generate User Event(user event=w1167, event data cluster=w1166) -> ()  [unwired: 2 in, 2 out]
      }
    }
    n320 = call "BypassAndLogErrors -- V2.vi"("Bypass Errors"=w195, "error in (no error)"=w194, "Log File Path"=w191) -> ("error out"=w193:errorcluster)  [unwired: 8 in]
  }
  n321 = while {
    tunnel: w8 -> [w1182]
    shift-right: [w1173] -> _
    shift-left: w2 -> [_]
    shift-right: [w1172] -> _
    shift-left: w5 -> [w1171]
    tunnel: w3 -> [w1169]
    i -> [w1177]
    stop <- FALSE ("Boolean") stop-if-true
    w1174 = u32 1000 ("milliseconds per cycle")
    w1180 = TRUE  # run dispatch loop
    w1176 = u32 6153 ("milliseconds per cycle")
    # "dispatch loop"
    n322 = Tick Count (ms)() -> (millisecond timer value=w1170:u32)
    n323 = Subtract(x=w1170, y=w1169) -> (x-y=w1168:u32)
    n324 = Equal To 0?(x=w1177) -> (x = 0?=w1185:bool)
    n325 = Divide(x=w1168, y=w1174) -> (x/y=w1173:dbl)
    "seconds" <- w1173
    n326 = case shown="True" w1185 {
      tunnel: w1171 -> [w1197 w1200]
      tunnel: [w1197 w1198] -> w1183
      frame False {
      }
      frame True {
        w1199 = "all: init" ("event data")
        n327 = Generate User Event(user event=w1200, event data cluster=w1199) -> (user event out=w1198:refnum<user-event>)  [unwired: 2 in, 1 out]
        n328 = call "sweep init checklist.vi"("action"=w1199) -> ()  [unwired: 10 in, 1 out]
      }
    }
    n329 = Wait (ms)(milliseconds to wait=w1176) -> ()  [unwired: 1 out]
    n330 = Divide(x=w1173, y=60) -> (x/y=→"minutes":dbl)
    n331 = Divide(x=w1176, y=w1174) -> (x/y=→"seconds per cycle":dbl)
    n332 = call "sweep init checklist.vi"("action"="test" ("event data")) -> ("result"=w1179:bool)  [unwired: 10 in]
    n333 = And(x=w1180, y=w1179) -> (x .and. y?=w1178:bool)
    n334 = case shown="True" w1178 {
      tunnel: w1183 -> [w1188 w1190]
      tunnel: w1182 -> [_ w1191]
      tunnel: [w1188 w1189] -> w1172
      frame False {
      }
      frame True {
        n335 = for {
          tunnel: w1191 -> [w1196] mode=indexing
          shift-right: [w1193] -> w1189
          shift-left: w1190 -> [w1192]
          n336 = Concatenate Strings(w1196, " check" ("event data")) -> (w1194:string)
          n337 = Generate User Event(user event=w1192, event data cluster=w1194) -> (user event out=w1193:refnum<user-event>)  [unwired: 2 in, 1 out]
        }
      }
    }
    "milliseconds per cycle" <- w1176
  }
  n338 = disable-structure shown="Disabled" {
    disable-tunnel: _ -> [w1201 _]
    frame Disabled {
      n339 = for {
        tunnel: w1201 -> [w1207]
        tunnel: i32[] [3, 4, 5, 6] -> [w1203] mode=indexing
        # "pid contro page"
        n340 = property on="Tab: everything" class="TabCtl (strict)"() -> ("Pages"=w1209:refnum<vi>[])  [unwired: 2 in, 2 out]
        n341 = Select(t=T40."Page Disabled & Grayed" ("Page Enabled State"), s=w1207, f=T40."Page Enabled" ("Page Enabled State")) -> (s? t:f=w1204:T40)
        n342 = Index Array(array=w1209, index=w1203) -> (element=w1208:refnum<vi>)
        n343 = property on="Property Node" class="Page"(reference=w1208, "PageEnb"=w1204) -> ()  [unwired: 1 in, 2 out]
      }
    }
    frame Enabled {
    }
  }
